vi "ExportMeasuresToHTML.vi"(8 "error in (no error)":errorcluster, 11 "Table in":refnum<vi>) -> (0 "error out":errorcluster)   [LabVIEW 2012]
uses:
  GlobalVariables/UserInfos.vi
  GlobalVariables/MeasureExportStrings.vi
  GlobalVariables/MachineInfos.vi
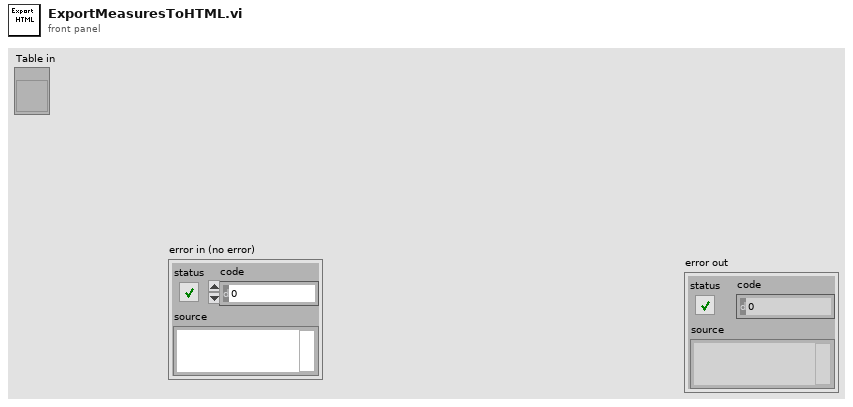
[diagram p1: front panel]
types:
  T1 = enum16{"open", "replace", "create", "open or create", "replace or create", "replace or create with confirmation"}
  T2 = cluster{"SerialNumber":string, "MachineName":string}
  T3 = cluster{"location":string, "Field":string, "Company":string, "Lab":string, "Operator":string, "Well":string, "Lat/Long":string, "Formation":string, "Country":string, "Client":string}
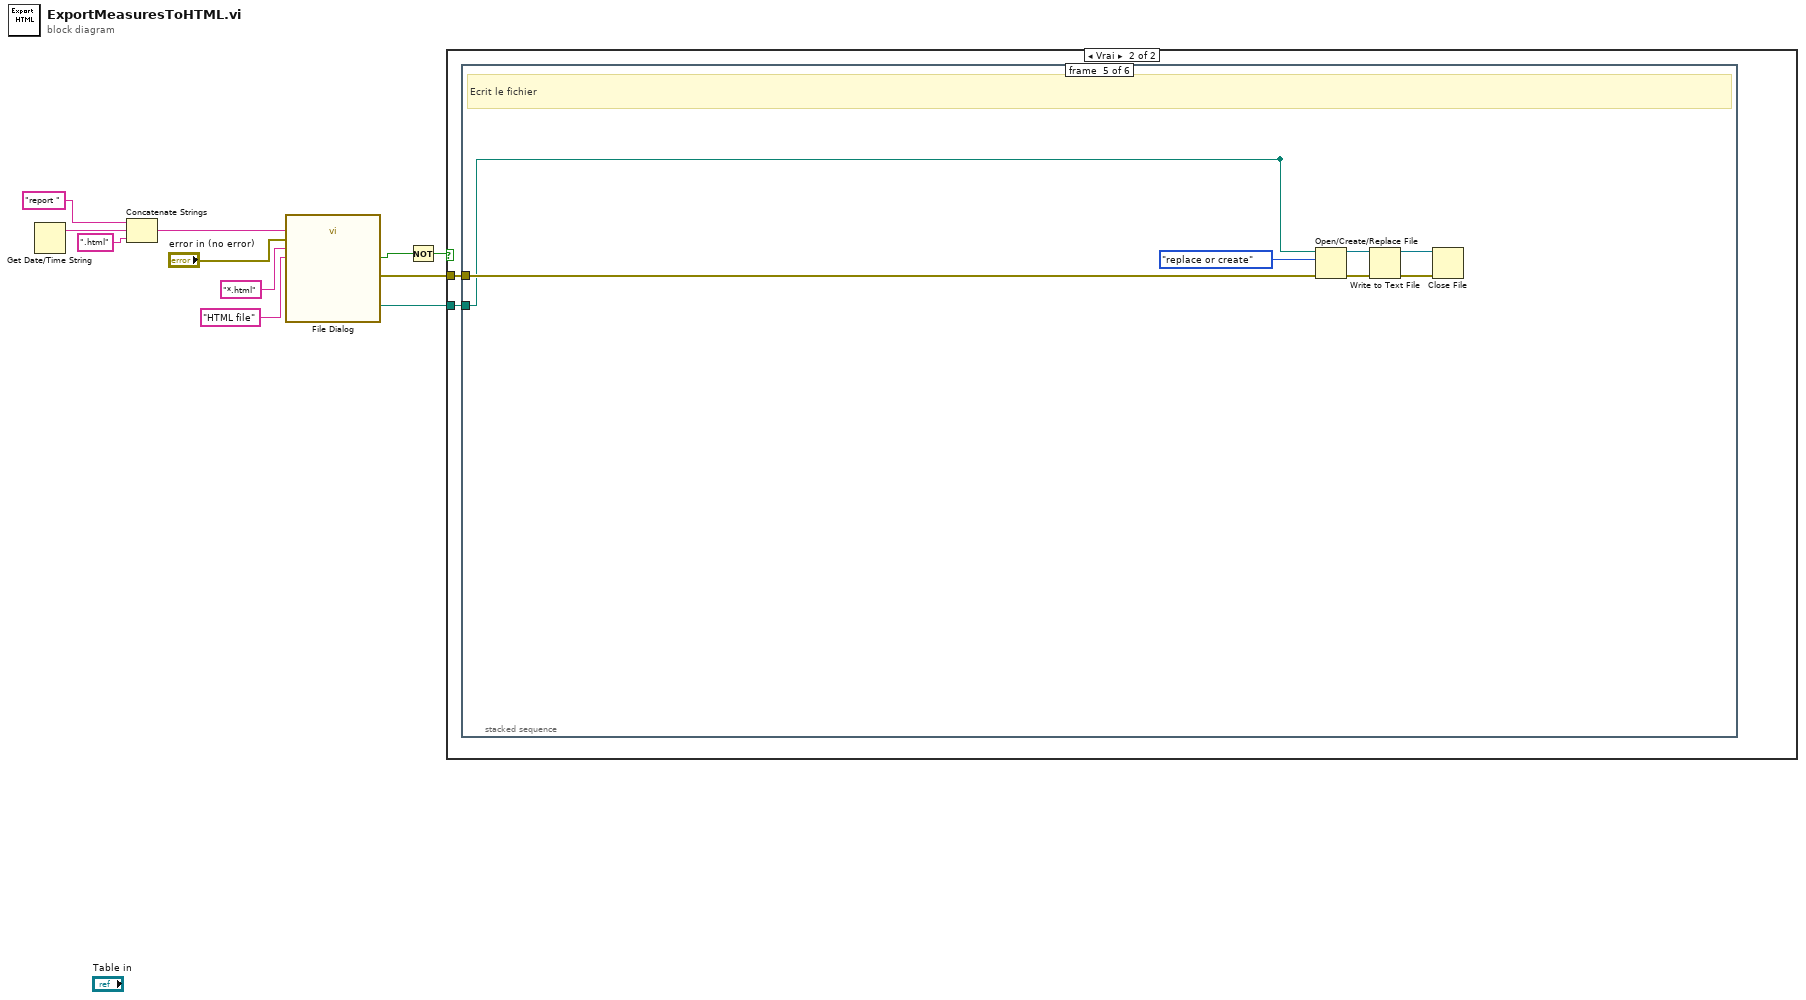
[diagram p0: block diagram]
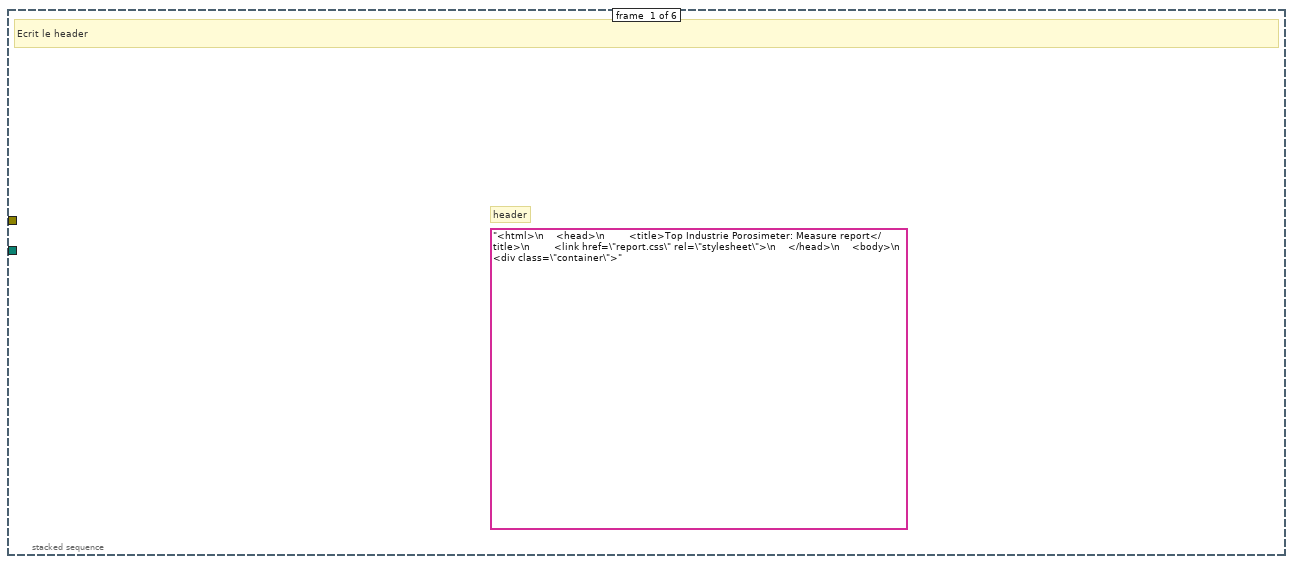
[diagram p3: hidden frame]
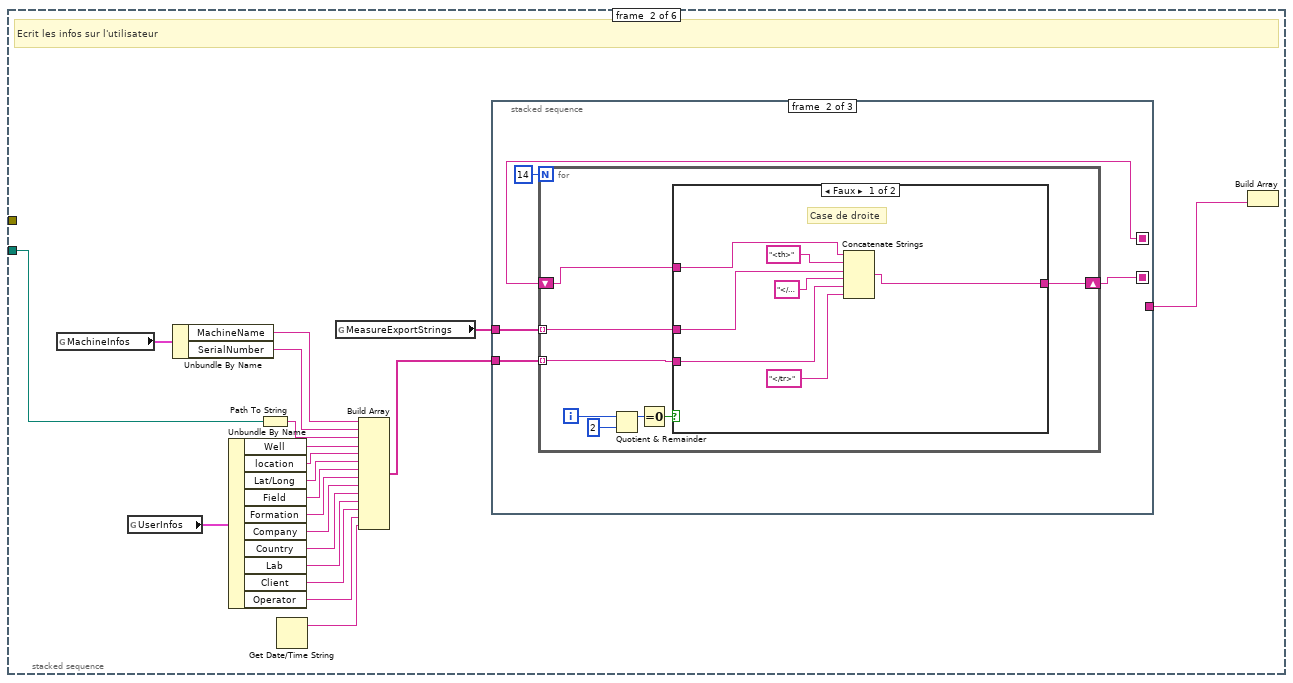
[diagram p4: hidden frame]
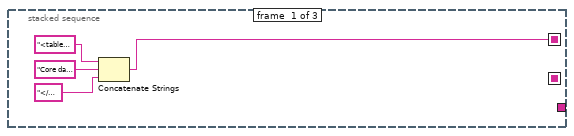
[diagram p5: hidden frame]
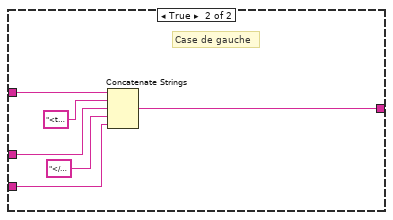
[diagram p6: hidden frame]
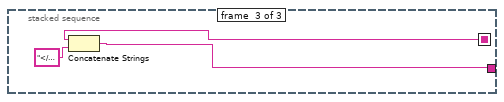
[diagram p7: hidden frame]
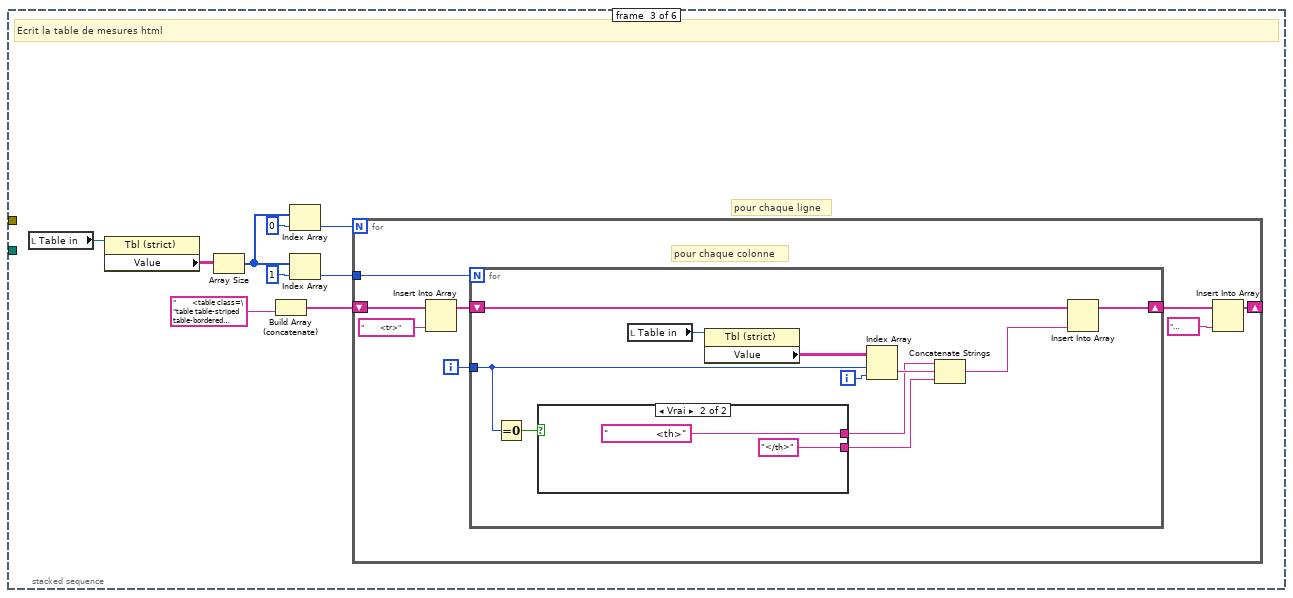
[diagram p8: hidden frame]
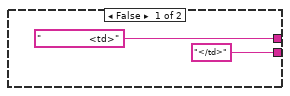
[diagram p9: hidden frame]
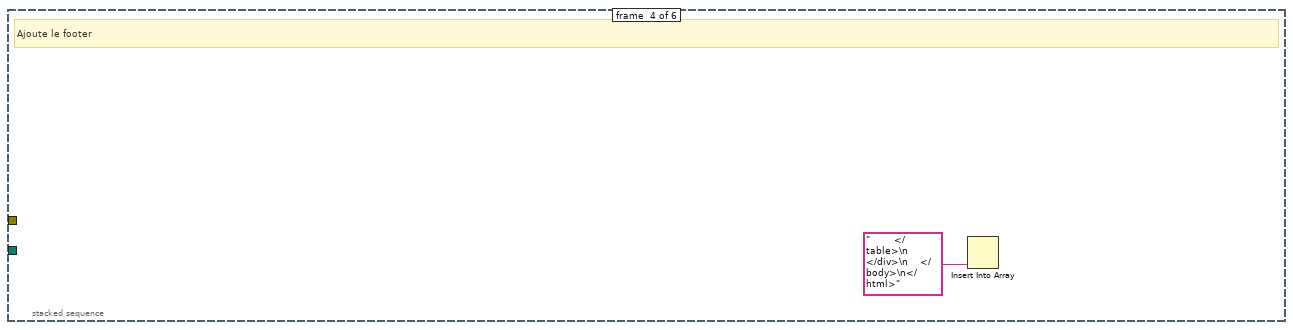
[diagram p10: hidden frame]
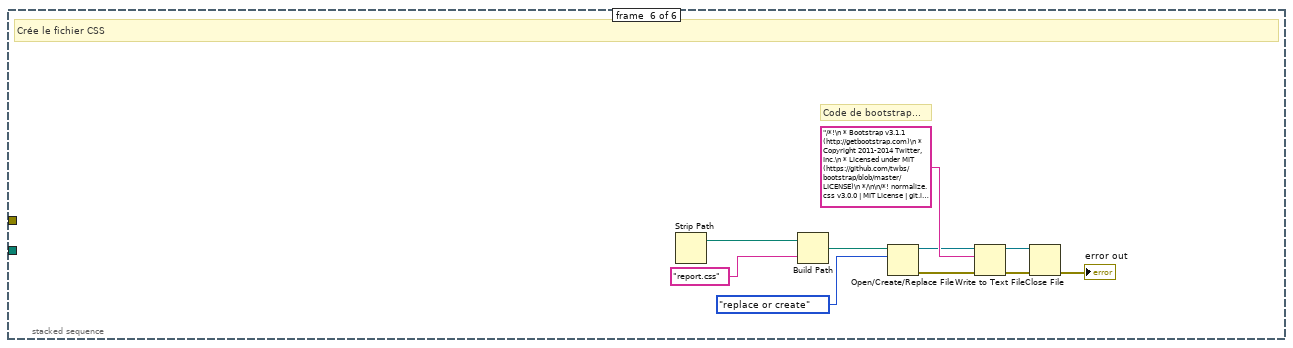
[diagram p11: hidden frame]
diagram:
  n1 = Get Date/Time String() -> (date string=w3:string)  [unwired: 3 in, 1 out]
  n2 = Concatenate Strings("report " ("string"), w3, ".html" ("string")) -> (w4:string)
  n3 = call "File Dialog"("default name"=w4, "error in"="error in (no error)", "pattern (all files)"="*.html", "pattern label"="HTML file") -> ("selected path"=w7:path, "cancelled"=w1:bool, "error out"=w8:errorcluster)  [unwired: 8 in, 1 out]
  n4 = Not(x=w1) -> (.not. x?=w2:bool)
  n5 = case shown="Vrai" w2 {
    tunnel: w8 -> [_ w13]
    tunnel: w7 -> [_ w12]
    frame False {
    }
    frame True {
      n6 = stacked-sequence {
        seq-local: ["<html>\n    <head>\n        <title>Top Industrie Porosimeter: Measure report</title>\n        <link href=\"report.css\" rel=\"stylesheet\">\n    </head>\n    <body>\n    <div class=\"container\">" _ _ _ _ _] -> [_ w36 _ _ _ _]
        seq-local: [_ w35 _ _ _ _] -> [_ _ w78 _ _ _]
        seq-local: [_ _ w77 _ _ _] -> [_ _ _ w105 _ _]
        seq-local: [_ _ _ w104 _ _] -> [_ _ _ _ w112 _]
        seq-local: [_ _ _ _ w113 _] -> [_ _ _ _ _ w120]
        seq-local: [_ _ _ _ w107 _] -> [_ _ _ _ _ w116]
        tunnel: w13 -> [_ _ _ _ w108 _]
        tunnel: w12 -> [_ w22 _ _ w107 _]
        frame #0 {
          # "header"
          # "Ecrit le header"
        }
        frame #1 {
          # "Ecrit les infos sur l'utilisateur"
          n7 = global read "MachineInfos.vi" "MachineInfos"() -> (w17:T2)
          n8 = global read "UserInfos.vi" "UserInfos"() -> (w34:T3)
          n9 = Unbundle By Name(w17) -> ("MachineName"=w16:string, "SerialNumber"=w15:string)
          n10 = Unbundle By Name(w34) -> ("Well"=w33:string, "location"=w32:string, "Lat/Long"=w31:string, "Field"=w30:string, "Formation"=w29:string, "Company"=w26:string, "Country"=w28:string, "Lab"=w27:string, "Client"=w25:string, "Operator"=w24:string)
          n11 = Path To String(path=w22) -> (string=w23:string)
          n12 = Get Date/Time String() -> (date string=w20:string)  [unwired: 3 in, 1 out]
          n13 = global read "MeasureExportStrings.vi" "MeasureExportStrings"() -> (w18:string[])
          n14 = Build Array(w16, w15, w23, w33, w32, w31, w30, w29, w26, w28, w27, w25, w24, w20) -> (w19:string[])
          n15 = stacked-sequence {
            seq-local: [w39 _ _] -> [_ w41 _]
            seq-local: [_ w42 _] -> [_ _ w68]
            tunnel: [_ _ w69] -> w21
            tunnel: w18 -> [_ w44 _]
            tunnel: w19 -> [_ w43 _]
            frame #0 {
              n16 = Concatenate Strings("<table class=\"table table-bordered table-condensed\">\n<tr>\n<td colspan=4> <h2 align=center>\n", "Core data report" ("string"), "</h2></td>\n</tr>" ("string")) -> (w39:string)
            }
            frame #1 {
              n17 = for {
                N: 14 -> [_]
                tunnel: w44 -> [w49] mode=indexing
                tunnel: w43 -> [w48] mode=indexing
                shift-right: [w47] -> w42
                shift-left: w41 -> [w46]
                i -> [w53]
                n18 = Quotient & Remainder(x=w53, y=2) -> (x-y*floor(x/y)=w50:i32)  [unwired: 1 out]
                n19 = Equal To 0?(x=w50) -> (x = 0?=w51:bool)
                n20 = case shown="Faux" w51 {
                  tunnel: w49 -> [w58 w65]
                  tunnel: w48 -> [w57 w63]
                  tunnel: [w55 w62] -> w47
                  tunnel: w46 -> [w54 w61]
                  frame False {
                    # "Case de droite"
                    n21 = Concatenate Strings(w54, "<th>", w58, "</th><td>", w57, "</tr>" ("string")) -> (w55:string)
                  }
                  frame True {
                    # "Case de gauche"
                    n22 = Concatenate Strings(w61, "<tr>\n<th>", w65, "</th><td>", w63) -> (w62:string)
                  }
                }
              }
            }
            frame #2 {
              n23 = Concatenate Strings(w68, "</table>\n" ("string")) -> (w69:string)
            }
          }
          n24 = Build Array(w36, w21) -> (w35:string[])
        }
        frame #2 {
          # "pour chaque ligne"
          # "Ecrit la table de mesures html"
          n25 = local read "Table in"() -> (w74:refnum<vi>)
          n26 = property on="Property Node" class="Tbl (strict)"(reference=w74) -> ("Value"=w75:string[][])  [unwired: 1 in, 2 out]
          n27 = Array Size(array=w75) -> (size(s)=w70:i32[])
          n28 = Build Array (concatenate)(w78, "        <table class=\"table table-striped table-bordered table-responsive\" >") -> (w80:string[])
          n29 = Index Array(array=w70, index=0) -> (element=w73:i32)
          n30 = Index Array(array=w70, index=1) -> (element=w72:i32)
          n31 = for {
            N: w73 -> [_]
            shift-right: [w88] -> w77
            shift-left: w80 -> [w87]
            tunnel: w72 -> [w86]
            i -> [w82]
            # "pour chaque colonne"
            n32 = Insert Into Array(array=w87, new element="        <tr>" ("new element/subarray")) -> (w84:string[])  [unwired: 1 in]
            n33 = for {
              N: w86 -> [_]
              shift-right: [w98] -> w85
              shift-left: w84 -> [w99]
              tunnel: w82 -> [w89]
              i -> [w91]
              n34 = Equal To 0?(x=w89) -> (x = 0?=w90:bool)
              n35 = case shown="Vrai" w90 {
                tunnel: ["</td>" "</th>"] -> w94
                tunnel: ["                <td>" "                <th>"] -> w92
                frame False {
                }
                frame True {
                }
              }
              n36 = local read "Table in"() -> (w95:refnum<vi>)
              n37 = property on="Property Node" class="Tbl (strict)"(reference=w95) -> ("Value"=w97:string[][])  [unwired: 1 in, 2 out]
              n38 = Index Array(array=w97, index (row)=w89, index (col)=w91) -> (element=w96:string)
              n39 = Concatenate Strings(w92, w96, w94) -> (w93:string)
              n40 = Insert Into Array(array=w99, new element=w93) -> (w98:string[])  [unwired: 1 in]
            }
            n41 = Insert Into Array(array=w85, new element="            </tr>") -> (w88:string[])  [unwired: 1 in]
          }
        }
        frame #3 {
          # "Ajoute le footer"
          n42 = Insert Into Array(array=w105, new element="        </table>\n        </div>\n    </body>\n</html>") -> (w104:string[])  [unwired: 1 in]
        }
        frame #4 {
          # "Ecrit le fichier"
          n43 = Open/Create/Replace File(file path (use dialog)=w107, error in=w108, operation (0:open)=T1."replace or create") -> (refnum out=w111:refnum<file>, error out=w114:errorcluster)  [unwired: 3 in, 1 out]
          n44 = Write to Text File(file (use dialog)=w111, text=w112, error in=w114) -> (refnum out=w109:refnum<file>, error out=w115:errorcluster)  [unwired: 1 in, 1 out]
          n45 = Close File(refnum=w109, error in=w115) -> (error out=w113:errorcluster)  [unwired: 1 out]
        }
        frame #5 {
          # "Code de bootstrap..."
          # "Crée le fichier CSS"
          n46 = Strip Path(path=w116) -> (stripped path=w119:path)  [unwired: 1 out]
          n47 = Build Path(base path=w119, name or relative path="report.css") -> (appended path=w117:path)
          n48 = Open/Create/Replace File(file path (use dialog)=w117, error in=w120, operation (0:open)=T1."replace or create") -> (refnum out=w125:refnum<file>, error out=w123:errorcluster)  [unwired: 3 in, 1 out]
          n49 = Write to Text File(file (use dialog)=w125, text="/*!\n * Bootstrap v3.1.1 (http://getbootstrap.com)\n * Copyright 2011-2014 Twitter, Inc.\n * Licensed under MIT (https://github.com/twbs/bootstrap/blob/master/LICENSE)\n */\n\n/*! normalize.css v3.0.0 | MIT License | git.io/normalize */\nhtml {\n  font-family: sans-serif;\n  -webkit-text-size-adjust: 100%;\n      -ms-text-size-adjust: 100%;\n}\nbody {\n  margin: 0;\n}\narticle,\naside,\ndetails,\nfigcaption,\nfigure,\nfooter,\nheader,\nhgroup,\nmain,\nnav,\nsection,\nsummary {\n  display: block;\n}\naudio,\ncanvas,\nprogress,\nvideo {\n  display: inline-block;\n  vertical-align: baseline;\n}\naudio:not([controls]) {\n  display: none;\n  height: 0;\n}\n[hidden],\ntemplate {\n  display: none;\n}\na {\n  background: transparent;\n}\na:active,\na:hover {\n  outline: 0;\n}\nabbr[title] {\n  border-bottom: 1px dotted;\n}\nb,\nstrong {\n  font-weight: bold;\n}\ndfn {\n  font-style: italic;\n}\nh1 {\n  margin: .67em 0;\n  font-size: 2em;\n}\nmark {\n  color: #000;\n  background: #ff0;\n}\nsmall {\n  font-size: 80%;\n}\nsub,\nsup {\n  position: relative;\n  font-size: 75%;\n  line-height: 0;\n  vertical-align: baseline;\n}\nsup {\n  top: -.5em;\n}\nsub {\n  bottom: -.25em;\n}\nimg {\n  border: 0;\n}\nsvg:not(:root) {\n  overflow: hidden;\n}\nfigure {\n  margin: 1em 40px;\n}\nhr {\n  height: 0;\n  -moz-box-sizing: content-box;\n       box-sizing: content-box;\n}\npre {\n  overflow: auto;\n}\ncode,\nkbd,\npre,\nsamp {\n  font-family: monospace, monospace;\n  font-size: 1em;\n}\nbutton,\ninput,\noptgroup,\nselect,\ntextarea {\n  margin: 0;\n  font: inherit;\n  color: inherit;\n}\nbutton {\n  overflow: visible;\n}\nbutton,\nselect {\n  text-transform: none;\n}\nbutton,\nhtml input[type=\"button\"],\ninput[type=\"reset\"],\ninput[type=\"submit\"] {\n  -webkit-appearance: button;\n  cursor: pointer;\n}\nbutton[disabled],\nhtml input[disabled] {\n  cursor: default;\n}\nbutton::-moz-focus-inner,\ninput::-moz-focus-inner {\n  padding: 0;\n  border: 0;\n}\ninput {\n  line-height: normal;\n}\ninput[type=\"checkbox\"],\ninput[type=\"radio\"] {\n  box-sizing: border-box;\n  padding: 0;\n}\ninput[type=\"number\"]::-webkit-inner-spin-button,\ninput[type=\"number\"]::-webkit-outer-spin-button {\n  height: auto;\n}\ninput[type=\"search\"] {\n  -webkit-box-sizing: content-box;\n     -moz-box-sizing: content-box;\n          box-sizing: content-box;\n  -webkit-appearance: textfield;\n}\ninput[type=\"search\"]::-webkit-search-cancel-button,\ninput[type=\"search\"]::-webkit-search-decoration {\n  -webkit-appearance: none;\n}\nfieldset {\n  padding: .35em .625em .75em;\n  margin: 0 2px;\n  border: 1px solid #c0c0c0;\n}\nlegend {\n  padding: 0;\n  border: 0;\n}\ntextarea {\n  overflow: auto;\n}\noptgroup {\n  font-weight: bold;\n}\ntable {\n  border-spacing: 0;\n  border-collapse: collapse;\n}\ntd,\nth {\n  padding: 0;\n}\n@media print {\n  * {\n    color: #000 !important;\n    text-shadow: none !important;\n    background: transparent !important;\n    box-shadow: none !important;\n  }\n  a,\n  a:visited {\n    text-decoration: underline;\n  }\n  a[href]:after {\n    content: \" (\" attr(href) \")\";\n  }\n  abbr[title]:after {\n    content: \" (\" attr(title) \")\";\n  }\n  a[href^=\"javascript:\"]:after,\n  a[href^=\"#\"]:after {\n    content: \"\";\n  }\n  pre,\n  blockquote {\n    border: 1px solid #999;\n\n    page-break-inside: avoid;\n  }\n  thead {\n    display: table-header-group;\n  }\n  tr,\n  img {\n    page-break-inside: avoid;\n  }\n  img {\n    max-width: 100% !important;\n  }\n  p,\n  h2,\n  h3 {\n    orphans: 3;\n    widows: 3;\n  }\n  h2,\n  h3 {\n    page-break-after: avoid;\n  }\n  select {\n    background: #fff !important;\n  }\n  .navbar {\n    display: none;\n  }\n  .table td,\n  .table th {\n    background-color: #fff !important;\n  }\n  .btn > .caret,\n  .dropup > .btn > .caret {\n    border-top-color: #000 !important;\n  }\n  .label {\n    border: 1px solid #000;\n  }\n  .table {\n    border-collapse: collapse !important;\n  }\n  .table-bordered th,\n  .table-bordered td {\n    border: 1px solid #ddd !important;\n  }\n}\n* {\n  -webkit-box-sizing: border-box;\n     -moz-box-sizing: border-box;\n          box-sizing: border-box;\n}\n*:before,\n*:after {\n  -webkit-box-sizing: border-box;\n     -moz-box-sizing: border-box;\n          box-sizing: border-box;\n}\nhtml {\n  font-size: 62.5%;\n\n  -webkit-tap-highlight-color: rgba(0, 0, 0, 0);\n}\nbody {\n  font-family: \"Helvetica Neue\", Helvetica, Arial, sans-serif;\n  font-size: 14px;\n  line-height: 1.42857143;\n  color: #333;\n  background-color: #fff;\n}\ninput,\nbutton,\nselect,\ntextarea {\n  font-family: inherit;\n  font-size: inherit;\n  line-height: inherit;\n}\na {\n  color: #428bca;\n  text-decoration: none;\n}\na:hover,\na:focus {\n  color: #2a6496;\n  text-decoration: underline;\n}\na:focus {\n  outline: thin dotted;\n  outline: 5px auto -webkit-focus-ring-color;\n  outline-offset: -2px;\n}\nfigure {\n  margin: 0;\n}\nimg {\n  vertical-align: middle;\n}\n.img-responsive,\n.thumbnail > img,\n.thumbnail a > img,\n.carousel-inner > .item > img,\n.carousel-inner > .item > a > img {\n  display: block;\n  max-width: 100%;\n  height: auto;\n}\n.img-rounded {\n  border-radius: 6px;\n}\n.img-thumbnail {\n  display: inline-block;\n  max-width: 100%;\n  height: auto;\n  padding: 4px;\n  line-height: 1.42857143;\n  background-color: #fff;\n  border: 1px solid #ddd;\n  border-radius: 4px;\n  -webkit-transition: all .2s ease-in-out;\n          transition: all .2s ease-in-out;\n}\n.img-circle {\n  border-radius: 50%;\n}\nhr {\n  margin-top: 20px;\n  margin-bottom: 20px;\n  border: 0;\n  border-top: 1px solid #eee;\n}\n.sr-only {\n  position: absolute;\n  width: 1px;\n  height: 1px;\n  padding: 0;\n  margin: -1px;\n  overflow: hidden;\n  clip: rect(0, 0, 0, 0);\n  border: 0;\n}\nh1,\nh2,\nh3,\nh4,\nh5,\nh6,\n.h1,\n.h2,\n.h3,\n.h4,\n.h5,\n.h6 {\n  font-family: inherit;\n  font-weight: 500;\n  line-height: 1.1;\n  color: inherit;\n}\nh1 small,\nh2 small,\nh3 small,\nh4 small,\nh5 small,\nh6 small,\n.h1 small,\n.h2 small,\n.h3 small,\n.h4 small,\n.h5 small,\n.h6 small,\nh1 .small,\nh2 .small,\nh3 .small,\nh4 .small,\nh5 .small,\nh6 .small,\n.h1 .small,\n.h2 .small,\n.h3 .small,\n.h4 .small,\n.h5 .small,\n.h6 .small {\n  font-weight: normal;\n  line-height: 1;\n  color: #999;\n}\nh1,\n.h1,\nh2,\n.h2,\nh3,\n.h3 {\n  margin-top: 20px;\n  margin-bottom: 10px;\n}\nh1 small,\n.h1 small,\nh2 small,\n.h2 small,\nh3 small,\n.h3 small,\nh1 .small,\n.h1 .small,\nh2 .small,\n.h2 .small,\nh3 .small,\n.h3 .small {\n  font-size: 65%;\n}\nh4,\n.h4,\nh5,\n.h5,\nh6,\n.h6 {\n  margin-top: 10px;\n  margin-bottom: 10px;\n}\nh4 small,\n.h4 small,\nh5 small,\n.h5 small,\nh6 small,\n.h6 small,\nh4 .small,\n.h4 .small,\nh5 .small,\n.h5 .small,\nh6 .small,\n.h6 .small {\n  font-size: 75%;\n}\nh1,\n.h1 {\n  font-size: 36px;\n}\nh2,\n.h2 {\n  font-size: 30px;\n}\nh3,\n.h3 {\n  font-size: 24px;\n}\nh4,\n.h4 {\n  font-size: 18px;\n}\nh5,\n.h5 {\n  font-size: 14px;\n}\nh6,\n.h6 {\n  font-size: 12px;\n}\np {\n  margin: 0 0 10px;\n}\n.lead {\n  margin-bottom: 20px;\n  font-size: 16px;\n  font-weight: 200;\n  line-height: 1.4;\n}\n@media (min-width: 768px) {\n  .lead {\n    font-size: 21px;\n  }\n}\nsmall,\n.small {\n  font-size: 85%;\n}\ncite {\n  font-style: normal;\n}\n.text-left {\n  text-align: left;\n}\n.text-right {\n  text-align: right;\n}\n.text-center {\n  text-align: center;\n}\n.text-justify {\n  text-align: justify;\n}\n.text-muted {\n  color: #999;\n}\n.text-primary {\n  color: #428bca;\n}\na.text-primary:hover {\n  color: #3071a9;\n}\n.text-success {\n  color: #3c763d;\n}\na.text-success:hover {\n  color: #2b542c;\n}\n.text-info {\n  color: #31708f;\n}\na.text-info:hover {\n  color: #245269;\n}\n.text-warning {\n  color: #8a6d3b;\n}\na.text-warning:hover {\n  color: #66512c;\n}\n.text-danger {\n  color: #a94442;\n}\na.text-danger:hover {\n  color: #843534;\n}\n.bg-primary {\n  color: #fff;\n  background-color: #428bca;\n}\na.bg-primary:hover {\n  background-color: #3071a9;\n}\n.bg-success {\n  background-color: #dff0d8;\n}\na.bg-success:hover {\n  background-color: #c1e2b3;\n}\n.bg-info {\n  background-color: #d9edf7;\n}\na.bg-info:hover {\n  background-color: #afd9ee;\n}\n.bg-warning {\n  background-color: #fcf8e3;\n}\na.bg-warning:hover {\n  background-color: #f7ecb5;\n}\n.bg-danger {\n  background-color: #f2dede;\n}\na.bg-danger:hover {\n  background-color: #e4b9b9;\n}\n.page-header {\n  padding-bottom: 9px;\n  margin: 40px 0 20px;\n  border-bottom: 1px solid #eee;\n}\nul,\nol {\n  margin-top: 0;\n  margin-bottom: 10px;\n}\nul ul,\nol ul,\nul ol,\nol ol {\n  margin-bottom: 0;\n}\n.list-unstyled {\n  padding-left: 0;\n  list-style: none;\n}\n.list-inline {\n  padding-left: 0;\n  margin-left: -5px;\n  list-style: none;\n}\n.list-inline > li {\n  display: inline-block;\n  padding-right: 5px;\n  padding-left: 5px;\n}\ndl {\n  margin-top: 0;\n  margin-bottom: 20px;\n}\ndt,\ndd {\n  line-height: 1.42857143;\n}\ndt {\n  font-weight: bold;\n}\ndd {\n  margin-left: 0;\n}\n@media (min-width: 768px) {\n  .dl-horizontal dt {\n    float: left;\n    width: 160px;\n    overflow: hidden;\n    clear: left;\n    text-align: right;\n    text-overflow: ellipsis;\n    white-space: nowrap;\n  }\n  .dl-horizontal dd {\n    margin-left: 180px;\n  }\n}\nabbr[title],\nabbr[data-original-title] {\n  cursor: help;\n  border-bottom: 1px dotted #999;\n}\n.initialism {\n  font-size: 90%;\n  text-transform: uppercase;\n}\nblockquote {\n  padding: 10px 20px;\n  margin: 0 0 20px;\n  font-size: 17.5px;\n  border-left: 5px solid #eee;\n}\nblockquote p:last-child,\nblockquote ul:last-child,\nblockquote ol:last-child {\n  margin-bottom: 0;\n}\nblockquote footer,\nblockquote small,\nblockquote .small {\n  display: block;\n  font-size: 80%;\n  line-height: 1.42857143;\n  color: #999;\n}\nblockquote footer:before,\nblockquote small:before,\nblockquote .small:before {\n  content: '\\2014 \\00A0';\n}\n.blockquote-reverse,\nblockquote.pull-right {\n  padding-right: 15px;\n  padding-left: 0;\n  text-align: right;\n  border-right: 5px solid #eee;\n  border-left: 0;\n}\n.blockquote-reverse footer:before,\nblockquote.pull-right footer:before,\n.blockquote-reverse small:before,\nblockquote.pull-right small:before,\n.blockquote-reverse .small:before,\nblockquote.pull-right .small:before {\n  content: '';\n}\n.blockquote-reverse footer:after,\nblockquote.pull-right footer:after,\n.blockquote-reverse small:after,\nblockquote.pull-right small:after,\n.blockquote-reverse .small:after,\nblockquote.pull-right .small:after {\n  content: '\\00A0 \\2014';\n}\nblockquote:before,\nblockquote:after {\n  content: \"\";\n}\naddress {\n  margin-bottom: 20px;\n  font-style: normal;\n  line-height: 1.42857143;\n}\ncode,\nkbd,\npre,\nsamp {\n  font-family: Menlo, Monaco, Consolas, \"Courier New\", monospace;\n}\ncode {\n  padding: 2px 4px;\n  font-size: 90%;\n  color: #c7254e;\n  white-space: nowrap;\n  background-color: #f9f2f4;\n  border-radius: 4px;\n}\nkbd {\n  padding: 2px 4px;\n  font-size: 90%;\n  color: #fff;\n  background-color: #333;\n  border-radius: 3px;\n  box-shadow: inset 0 -1px 0 rgba(0, 0, 0, .25);\n}\npre {\n  display: block;\n  padding: 9.5px;\n  margin: 0 0 10px;\n  font-size: 13px;\n  line-height: 1.42857143;\n  color: #333;\n  word-break: break-all;\n  word-wrap: break-word;\n  background-color: #f5f5f5;\n  border: 1px solid #ccc;\n  border-radius: 4px;\n}\npre code {\n  padding: 0;\n  font-size: inherit;\n  color: inherit;\n  white-space: pre-wrap;\n  background-color: transparent;\n  border-radius: 0;\n}\n.pre-scrollable {\n  max-height: 340px;\n  overflow-y: scroll;\n}\n.container {\n  padding-right: 15px;\n  padding-left: 15px;\n  margin-right: auto;\n  margin-left: auto;\n}\n@media (min-width: 768px) {\n  .container {\n    width: 750px;\n  }\n}\n@media (min-width: 992px) {\n  .container {\n    width: 970px;\n  }\n}\n@media (min-width: 1200px) {\n  .container {\n    width: 1170px;\n  }\n}\n.container-fluid {\n  padding-right: 15px;\n  padding-left: 15px;\n  margin-right: auto;\n  margin-left: auto;\n}\n.row {\n  margin-right: -15px;\n  margin-left: -15px;\n}\n.col-xs-1, .col-sm-1, .col-md-1, .col-lg-1, .col-xs-2, .col-sm-2, .col-md-2, .col-lg-2, .col-xs-3, .col-sm-3, .col-md-3, .col-lg-3, .col-xs-4, .col-sm-4, .col-md-4, .col-lg-4, .col-xs-5, .col-sm-5, .col-md-5, .col-lg-5, .col-xs-6, .col-sm-6, .col-md-6, .col-lg-6, .col-xs-7, .col-sm-7, .col-md-7, .col-lg-7, .col-xs-8, .col-sm-8, .col-md-8, .col-lg-8, .col-xs-9, .col-sm-9, .col-md-9, .col-lg-9, .col-xs-10, .col-sm-10, .col-md-10, .col-lg-10, .col-xs-11, .col-sm-11, .col-md-11, .col-lg-11, .col-xs-12, .col-sm-12, .col-md-12, .col-lg-12 {\n  position: relative;\n  min-height: 1px;\n  padding-right: 15px;\n  padding-left: 15px;\n}\n.col-xs-1, .col-xs-2, .col-xs-3, .col-xs-4, .col-xs-5, .col-xs-6, .col-xs-7, .col-xs-8, .col-xs-9, .col-xs-10, .col-xs-11, .col-xs-12 {\n  float: left;\n}\n.col-xs-12 {\n  width: 100%;\n}\n.col-xs-11 {\n  width: 91.66666667%;\n}\n.col-xs-10 {\n  width: 83.33333333%;\n}\n.col-xs-9 {\n  width: 75%;\n}\n.col-xs-8 {\n  width: 66.66666667%;\n}\n.col-xs-7 {\n  width: 58.33333333%;\n}\n.col-xs-6 {\n  width: 50%;\n}\n.col-xs-5 {\n  width: 41.66666667%;\n}\n.col-xs-4 {\n  width: 33.33333333%;\n}\n.col-xs-3 {\n  width: 25%;\n}\n.col-xs-2 {\n  width: 16.66666667%;\n}\n.col-xs-1 {\n  width: 8.33333333%;\n}\n.col-xs-pull-12 {\n  right: 100%;\n}\n.col-xs-pull-11 {\n  right: 91.66666667%;\n}\n.col-xs-pull-10 {\n  right: 83.33333333%;\n}\n.col-xs-pull-9 {\n  right: 75%;\n}\n.col-xs-pull-8 {\n  right: 66.66666667%;\n}\n.col-xs-pull-7 {\n  right: 58.33333333%;\n}\n.col-xs-pull-6 {\n  right: 50%;\n}\n.col-xs-pull-5 {\n  right: 41.66666667%;\n}\n.col-xs-pull-4 {\n  right: 33.33333333%;\n}\n.col-xs-pull-3 {\n  right: 25%;\n}\n.col-xs-pull-2 {\n  right: 16.66666667%;\n}\n.col-xs-pull-1 {\n  right: 8.33333333%;\n}\n.col-xs-pull-0 {\n  right: 0;\n}\n.col-xs-push-12 {\n  left: 100%;\n}\n.col-xs-push-11 {\n  left: 91.66666667%;\n}\n.col-xs-push-10 {\n  left: 83.33333333%;\n}\n.col-xs-push-9 {\n  left: 75%;\n}\n.col-xs-push-8 {\n  left: 66.66666667%;\n}\n.col-xs-push-7 {\n  left: 58.33333333%;\n}\n.col-xs-push-6 {\n  left: 50%;\n}\n.col-xs-push-5 {\n  left: 41.66666667%;\n}\n.col-xs-push-4 {\n  left: 33.33333333%;\n}\n.col-xs-push-3 {\n  left: 25%;\n}\n.col-xs-push-2 {\n  left: 16.66666667%;\n}\n.col-xs-push-1 {\n  left: 8.33333333%;\n}\n.col-xs-push-0 {\n  left: 0;\n}\n.col-xs-offset-12 {\n  margin-left: 100%;\n}\n.col-xs-offset-11 {\n  margin-left: 91.66666667%;\n}\n.col-xs-offset-10 {\n  margin-left: 83.33333333%;\n}\n.col-xs-offset-9 {\n  margin-left: 75%;\n}\n.col-xs-offset-8 {\n  margin-left: 66.66666667%;\n}\n.col-xs-offset-7 {\n  margin-left: 58.33333333%;\n}\n.col-xs-offset-6 {\n  margin-left: 50%;\n}\n.col-xs-offset-5 {\n  margin-left: 41.66666667%;\n}\n.col-xs-offset-4 {\n  margin-left: 33.33333333%;\n}\n.col-xs-offset-3 {\n  margin-left: 25%;\n}\n.col-xs-offset-2 {\n  margin-left: 16.66666667%;\n}\n.col-xs-offset-1 {\n  margin-left: 8.33333333%;\n}\n.col-xs-offset-0 {\n  margin-left: 0;\n}\n@media (min-width: 768px) {\n  .col-sm-1, .col-sm-2, .col-sm-3, .col-sm-4, .col-sm-5, .col-sm-6, .col-sm-7, .col-sm-8, .col-sm-9, .col-sm-10, .col-sm-11, .col-sm-12 {\n    float: left;\n  }\n  .col-sm-12 {\n    width: 100%;\n  }\n  .col-sm-11 {\n    width: 91.66666667%;\n  }\n  .col-sm-10 {\n    width: 83.33333333%;\n  }\n  .col-sm-9 {\n    width: 75%;\n  }\n  .col-sm-8 {\n    width: 66.66666667%;\n  }\n  .col-sm-7 {\n    width: 58.33333333%;\n  }\n  .col-sm-6 {\n    width: 50%;\n  }\n  .col-sm-5 {\n    width: 41.66666667%;\n  }\n  .col-sm-4 {\n    width: 33.33333333%;\n  }\n  .col-sm-3 {\n    width: 25%;\n  }\n  .col-sm-2 {\n    width: 16.66666667%;\n  }\n  .col-sm-1 {\n    width: 8.33333333%;\n  }\n  .col-sm-pull-12 {\n    right: 100%;\n  }\n  .col-sm-pull-11 {\n    right: 91.66666667%;\n  }\n  .col-sm-pull-10 {\n    right: 83.33333333%;\n  }\n  .col-sm-pull-9 {\n    right: 75%;\n  }\n  .col-sm-pull-8 {\n    right: 66.66666667%;\n  }\n  .col-sm-pull-7 {\n    right: 58.33333333%;\n  }\n  .col-sm-pull-6 {\n    right: 50%;\n  }\n  .col-sm-pull-5 {\n    right: 41.66666667%;\n  }\n  .col-sm-pull-4 {\n    right: 33.33333333%;\n  }\n  .col-sm-pull-3 {\n    right: 25%;\n  }\n  .col-sm-pull-2 {\n    right: 16.66666667%;\n  }\n  .col-sm-pull-1 {\n    right: 8.33333333%;\n  }\n  .col-sm-pull-0 {\n    right: 0;\n  }\n  .col-sm-push-12 {\n    left: 100%;\n  }\n  .col-sm-push-11 {\n    left: 91.66666667%;\n  }\n  .col-sm-push-10 {\n    left: 83.33333333%;\n  }\n  .col-sm-push-9 {\n    left: 75%;\n  }\n  .col-sm-push-8 {\n    left: 66.66666667%;\n  }\n  .col-sm-push-7 {\n    left: 58.33333333%;\n  }\n  .col-sm-push-6 {\n    left: 50%;\n  }\n  .col-sm-push-5 {\n    left: 41.66666667%;\n  }\n  .col-sm-push-4 {\n    left: 33.33333333%;\n  }\n  .col-sm-push-3 {\n    left: 25%;\n  }\n  .col-sm-push-2 {\n    left: 16.66666667%;\n  }\n  .col-sm-push-1 {\n    left: 8.33333333%;\n  }\n  .col-sm-push-0 {\n    left: 0;\n  }\n  .col-sm-offset-12 {\n    margin-left: 100%;\n  }\n  .col-sm-offset-11 {\n    margin-left: 91.66666667%;\n  }\n  .col-sm-offset-10 {\n    margin-left: 83.33333333%;\n  }\n  .col-sm-offset-9 {\n    margin-left: 75%;\n  }\n  .col-sm-offset-8 {\n    margin-left: 66.66666667%;\n  }\n  .col-sm-offset-7 {\n    margin-left: 58.33333333%;\n  }\n  .col-sm-offset-6 {\n    margin-left: 50%;\n  }\n  .col-sm-offset-5 {\n    margin-left: 41.66666667%;\n  }\n  .col-sm-offset-4 {\n    margin-left: 33.33333333%;\n  }\n  .col-sm-offset-3 {\n    margin-left: 25%;\n  }\n  .col-sm-offset-2 {\n    margin-left: 16.66666667%;\n  }\n  .col-sm-offset-1 {\n    margin-left: 8.33333333%;\n  }\n  .col-sm-offset-0 {\n    margin-left: 0;\n  }\n}\n@media (min-width: 992px) {\n  .col-md-1, .col-md-2, .col-md-3, .col-md-4, .col-md-5, .col-md-6, .col-md-7, .col-md-8, .col-md-9, .col-md-10, .col-md-11, .col-md-12 {\n    float: left;\n  }\n  .col-md-12 {\n    width: 100%;\n  }\n  .col-md-11 {\n    width: 91.66666667%;\n  }\n  .col-md-10 {\n    width: 83.33333333%;\n  }\n  .col-md-9 {\n    width: 75%;\n  }\n  .col-md-8 {\n    width: 66.66666667%;\n  }\n  .col-md-7 {\n    width: 58.33333333%;\n  }\n  .col-md-6 {\n    width: 50%;\n  }\n  .col-md-5 {\n    width: 41.66666667%;\n  }\n  .col-md-4 {\n    width: 33.33333333%;\n  }\n  .col-md-3 {\n    width: 25%;\n  }\n  .col-md-2 {\n    width: 16.66666667%;\n  }\n  .col-md-1 {\n    width: 8.33333333%;\n  }\n  .col-md-pull-12 {\n    right: 100%;\n  }\n  .col-md-pull-11 {\n    right: 91.66666667%;\n  }\n  .col-md-pull-10 {\n    right: 83.33333333%;\n  }\n  .col-md-pull-9 {\n    right: 75%;\n  }\n  .col-md-pull-8 {\n    right: 66.66666667%;\n  }\n  .col-md-pull-7 {\n    right: 58.33333333%;\n  }\n  .col-md-pull-6 {\n    right: 50%;\n  }\n  .col-md-pull-5 {\n    right: 41.66666667%;\n  }\n  .col-md-pull-4 {\n    right: 33.33333333%;\n  }\n  .col-md-pull-3 {\n    right: 25%;\n  }\n  .col-md-pull-2 {\n    right: 16.66666667%;\n  }\n  .col-md-pull-1 {\n    right: 8.33333333%;\n  }\n  .col-md-pull-0 {\n    right: 0;\n  }\n  .col-md-push-12 {\n    left: 100%;\n  }\n  .col-md-push-11 {\n    left: 91.66666667%;\n  }\n  .col-md-push-10 {\n    left: 83.33333333%;\n  }\n  .col-md-push-9 {\n    left: 75%;\n  }\n  .col-md-push-8 {\n    left: 66.66666667%;\n  }\n  .col-md-push-7 {\n    left: 58.33333333%;\n  }\n  .col-md-push-6 {\n    left: 50%;\n  }\n  .col-md-push-5 {\n    left: 41.66666667%;\n  }\n  .col-md-push-4 {\n    left: 33.33333333%;\n  }\n  .col-md-push-3 {\n    left: 25%;\n  }\n  .col-md-push-2 {\n    left: 16.66666667%;\n  }\n  .col-md-push-1 {\n    left: 8.33333333%;\n  }\n  .col-md-push-0 {\n    left: 0;\n  }\n  .col-md-offset-12 {\n    margin-left: 100%;\n  }\n  .col-md-offset-11 {\n    margin-left: 91.66666667%;\n  }\n  .col-md-offset-10 {\n    margin-left: 83.33333333%;\n  }\n  .col-md-offset-9 {\n    margin-left: 75%;\n  }\n  .col-md-offset-8 {\n    margin-left: 66.66666667%;\n  }\n  .col-md-offset-7 {\n    margin-left: 58.33333333%;\n  }\n  .col-md-offset-6 {\n    margin-left: 50%;\n  }\n  .col-md-offset-5 {\n    margin-left: 41.66666667%;\n  }\n  .col-md-offset-4 {\n    margin-left: 33.33333333%;\n  }\n  .col-md-offset-3 {\n    margin-left: 25%;\n  }\n  .col-md-offset-2 {\n    margin-left: 16.66666667%;\n  }\n  .col-md-offset-1 {\n    margin-left: 8.33333333%;\n  }\n  .col-md-offset-0 {\n    margin-left: 0;\n  }\n}\n@media (min-width: 1200px) {\n  .col-lg-1, .col-lg-2, .col-lg-3, .col-lg-4, .col-lg-5, .col-lg-6, .col-lg-7, .col-lg-8, .col-lg-9, .col-lg-10, .col-lg-11, .col-lg-12 {\n    float: left;\n  }\n  .col-lg-12 {\n    width: 100%;\n  }\n  .col-lg-11 {\n    width: 91.66666667%;\n  }\n  .col-lg-10 {\n    width: 83.33333333%;\n  }\n  .col-lg-9 {\n    width: 75%;\n  }\n  .col-lg-8 {\n    width: 66.66666667%;\n  }\n  .col-lg-7 {\n    width: 58.33333333%;\n  }\n  .col-lg-6 {\n    width: 50%;\n  }\n  .col-lg-5 {\n    width: 41.66666667%;\n  }\n  .col-lg-4 {\n    width: 33.33333333%;\n  }\n  .col-lg-3 {\n    width: 25%;\n  }\n  .col-lg-2 {\n    width: 16.66666667%;\n  }\n  .col-lg-1 {\n    width: 8.33333333%;\n  }\n  .col-lg-pull-12 {\n    right: 100%;\n  }\n  .col-lg-pull-11 {\n    right: 91.66666667%;\n  }\n  .col-lg-pull-10 {\n    right: 83.33333333%;\n  }\n  .col-lg-pull-9 {\n    right: 75%;\n  }\n  .col-lg-pull-8 {\n    right: 66.66666667%;\n  }\n  .col-lg-pull-7 {\n    right: 58.33333333%;\n  }\n  .col-lg-pull-6 {\n    right: 50%;\n  }\n  .col-lg-pull-5 {\n    right: 41.66666667%;\n  }\n  .col-lg-pull-4 {\n    right: 33.33333333%;\n  }\n  .col-lg-pull-3 {\n    right: 25%;\n  }\n  .col-lg-pull-2 {\n    right: 16.66666667%;\n  }\n  .col-lg-pull-1 {\n    right: 8.33333333%;\n  }\n  .col-lg-pull-0 {\n    right: 0;\n  }\n  .col-lg-push-12 {\n    left: 100%;\n  }\n  .col-lg-push-11 {\n    left: 91.66666667%;\n  }\n  .col-lg-push-10 {\n    left: 83.33333333%;\n  }\n  .col-lg-push-9 {\n    left: 75%;\n  }\n  .col-lg-push-8 {\n    left: 66.66666667%;\n  }\n  .col-lg-push-7 {\n    left: 58.33333333%;\n  }\n  .col-lg-push-6 {\n    left: 50%;\n  }\n  .col-lg-push-5 {\n    left: 41.66666667%;\n  }\n  .col-lg-push-4 {\n    left: 33.33333333%;\n  }\n  .col-lg-push-3 {\n    left: 25%;\n  }\n  .col-lg-push-2 {\n    left: 16.66666667%;\n  }\n  .col-lg-push-1 {\n    left: 8.33333333%;\n  }\n  .col-lg-push-0 {\n    left: 0;\n  }\n  .col-lg-offset-12 {\n    margin-left: 100%;\n  }\n  .col-lg-offset-11 {\n    margin-left: 91.66666667%;\n  }\n  .col-lg-offset-10 {\n    margin-left: 83.33333333%;\n  }\n  .col-lg-offset-9 {\n    margin-left: 75%;\n  }\n  .col-lg-offset-8 {\n    margin-left: 66.66666667%;\n  }\n  .col-lg-offset-7 {\n    margin-left: 58.33333333%;\n  }\n  .col-lg-offset-6 {\n    margin-left: 50%;\n  }\n  .col-lg-offset-5 {\n    margin-left: 41.66666667%;\n  }\n  .col-lg-offset-4 {\n    margin-left: 33.33333333%;\n  }\n  .col-lg-offset-3 {\n    margin-left: 25%;\n  }\n  .col-lg-offset-2 {\n    margin-left: 16.66666667%;\n  }\n  .col-lg-offset-1 {\n    margin-left: 8.33333333%;\n  }\n  .col-lg-offset-0 {\n    margin-left: 0;\n  }\n}\ntable {\n  max-width: 100%;\n  background-color: transparent;\n}\nth {\n  text-align: left;\n}\n.table {\n  width: 100%;\n  margin-bottom: 20px;\n}\n.table > thead > tr > th,\n.table > tbody > tr > th,\n.table > tfoot > tr > th,\n.table > thead > tr > td,\n.table > tbody > tr > td,\n.table > tfoot > tr > td {\n  padding: 2px;\n  line-height: 1.42857143;\n  vertical-align: top;\n  border-top: 1px solid #ddd;\n}\n.table > thead > tr > th {\n  vertical-align: bottom;\n  border-bottom: 2px solid #ddd;\n}\n.table > caption + thead > tr:first-child > th,\n.table > colgroup + thead > tr:first-child > th,\n.table > thead:first-child > tr:first-child > th,\n.table > caption + thead > tr:first-child > td,\n.table > colgroup + thead > tr:first-child > td,\n.table > thead:first-child > tr:first-child > td {\n  border-top: 0;\n}\n.table > tbody + tbody {\n  border-top: 2px solid #ddd;\n}\n.table .table {\n  background-color: #fff;\n}\n.table-condensed > thead > tr > th,\n.table-condensed > tbody > tr > th,\n.table-condensed > tfoot > tr > th,\n.table-condensed > thead > tr > td,\n.table-condensed > tbody > tr > td,\n.table-condensed > tfoot > tr > td {\n  padding: 2px;\n}\n.table-bordered {\n  border: 1px solid #ddd;\n}\n.table-bordered > thead > tr > th,\n.table-bordered > tbody > tr > th,\n.table-bordered > tfoot > tr > th,\n.table-bordered > thead > tr > td,\n.table-bordered > tbody > tr > td,\n.table-bordered > tfoot > tr > td {\n  border: 1px solid #ddd;\n}\n.table-bordered > thead > tr > th,\n.table-bordered > thead > tr > td {\n  border-bottom-width: 2px;\n}\n.table-striped > tbody > tr:nth-child(odd) > td,\n.table-striped > tbody > tr:nth-child(odd) > th {\n  background-color: #f9f9f9;\n}\n.table-hover > tbody > tr:hover > td,\n.table-hover > tbody > tr:hover > th {\n  background-color: #f5f5f5;\n}\ntable col[class*=\"col-\"] {\n  position: static;\n  display: table-column;\n  float: none;\n}\ntable td[class*=\"col-\"],\ntable th[class*=\"col-\"] {\n  position: static;\n  display: table-cell;\n  float: none;\n}\n.table > thead > tr > td.active,\n.table > tbody > tr > td.active,\n.table > tfoot > tr > td.active,\n.table > thead > tr > th.active,\n.table > tbody > tr > th.active,\n.table > tfoot > tr > th.active,\n.table > thead > tr.active > td,\n.table > tbody > tr.active > td,\n.table > tfoot > tr.active > td,\n.table > thead > tr.active > th,\n.table > tbody > tr.active > th,\n.table > tfoot > tr.active > th {\n  background-color: #f5f5f5;\n}\n.table-hover > tbody > tr > td.active:hover,\n.table-hover > tbody > tr > th.active:hover,\n.table-hover > tbody > tr.active:hover > td,\n.table-hover > tbody > tr.active:hover > th {\n  background-color: #e8e8e8;\n}\n.table > thead > tr > td.success,\n.table > tbody > tr > td.success,\n.table > tfoot > tr > td.success,\n.table > thead > tr > th.success,\n.table > tbody > tr > th.success,\n.table > tfoot > tr > th.success,\n.table > thead > tr.success > td,\n.table > tbody > tr.success > td,\n.table > tfoot > tr.success > td,\n.table > thead > tr.success > th,\n.table > tbody > tr.success > th,\n.table > tfoot > tr.success > th {\n  background-color: #dff0d8;\n}\n.table-hover > tbody > tr > td.success:hover,\n.table-hover > tbody > tr > th.success:hover,\n.table-hover > tbody > tr.success:hover > td,\n.table-hover > tbody > tr.success:hover > th {\n  background-color: #d0e9c6;\n}\n.table > thead > tr > td.info,\n.table > tbody > tr > td.info,\n.table > tfoot > tr > td.info,\n.table > thead > tr > th.info,\n.table > tbody > tr > th.info,\n.table > tfoot > tr > th.info,\n.table > thead > tr.info > td,\n.table > tbody > tr.info > td,\n.table > tfoot > tr.info > td,\n.table > thead > tr.info > th,\n.table > tbody > tr.info > th,\n.table > tfoot > tr.info > th {\n  background-color: #d9edf7;\n}\n.table-hover > tbody > tr > td.info:hover,\n.table-hover > tbody > tr > th.info:hover,\n.table-hover > tbody > tr.info:hover > td,\n.table-hover > tbody > tr.info:hover > th {\n  background-color: #c4e3f3;\n}\n.table > thead > tr > td.warning,\n.table > tbody > tr > td.warning,\n.table > tfoot > tr > td.warning,\n.table > thead > tr > th.warning,\n.table > tbody > tr > th.warning,\n.table > tfoot > tr > th.warning,\n.table > thead > tr.warning > td,\n.table > tbody > tr.warning > td,\n.table > tfoot > tr.warning > td,\n.table > thead > tr.warning > th,\n.table > tbody > tr.warning > th,\n.table > tfoot > tr.warning > th {\n  background-color: #fcf8e3;\n}\n.table-hover > tbody > tr > td.warning:hover,\n.table-hover > tbody > tr > th.warning:hover,\n.table-hover > tbody > tr.warning:hover > td,\n.table-hover > tbody > tr.warning:hover > th {\n  background-color: #faf2cc;\n}\n.table > thead > tr > td.danger,\n.table > tbody > tr > td.danger,\n.table > tfoot > tr > td.danger,\n.table > thead > tr > th.danger,\n.table > tbody > tr > th.danger,\n.table > tfoot > tr > th.danger,\n.table > thead > tr.danger > td,\n.table > tbody > tr.danger > td,\n.table > tfoot > tr.danger > td,\n.table > thead > tr.danger > th,\n.table > tbody > tr.danger > th,\n.table > tfoot > tr.danger > th {\n  background-color: #f2dede;\n}\n.table-hover > tbody > tr > td.danger:hover,\n.table-hover > tbody > tr > th.danger:hover,\n.table-hover > tbody > tr.danger:hover > td,\n.table-hover > tbody > tr.danger:hover > th {\n  background-color: #ebcccc;\n}\n@media (max-width: 767px) {\n  .table-responsive {\n    width: 100%;\n    margin-bottom: 15px;\n    overflow-x: scroll;\n    overflow-y: hidden;\n    -webkit-overflow-scrolling: touch;\n    -ms-overflow-style: -ms-autohiding-scrollbar;\n    border: 1px solid #ddd;\n  }\n  .table-responsive > .table {\n    margin-bottom: 0;\n  }\n  .table-responsive > .table > thead > tr > th,\n  .table-responsive > .table > tbody > tr > th,\n  .table-responsive > .table > tfoot > tr > th,\n  .table-responsive > .table > thead > tr > td,\n  .table-responsive > .table > tbody > tr > td,\n  .table-responsive > .table > tfoot > tr > td {\n    white-space: nowrap;\n  }\n  .table-responsive > .table-bordered {\n    border: 0;\n  }\n  .table-responsive > .table-bordered > thead > tr > th:first-child,\n  .table-responsive > .table-bordered > tbody > tr > th:first-child,\n  .table-responsive > .table-bordered > tfoot > tr > th:first-child,\n  .table-responsive > .table-bordered > thead > tr > td:first-child,\n  .table-responsive > .table-bordered > tbody > tr > td:first-child,\n  .table-responsive > .table-bordered > tfoot > tr > td:first-child {\n    border-left: 0;\n  }\n  .table-responsive > .table-bordered > thead > tr > th:last-child,\n  .table-responsive > .table-bordered > tbody > tr > th:last-child,\n  .table-responsive > .table-bordered > tfoot > tr > th:last-child,\n  .table-responsive > .table-bordered > thead > tr > td:last-child,\n  .table-responsive > .table-bordered > tbody > tr > td:last-child,\n  .table-responsive > .table-bordered > tfoot > tr > td:last-child {\n    border-right: 0;\n  }\n  .table-responsive > .table-bordered > tbody > tr:last-child > th,\n  .table-responsive > .table-bordered > tfoot > tr:last-child > th,\n  .table-responsive > .table-bordered > tbody > tr:last-child > td,\n  .table-responsive > .table-bordered > tfoot > tr:last-child > td {\n    border-bottom: 0;\n  }\n}\nfieldset {\n  min-width: 0;\n  padding: 0;\n  margin: 0;\n  border: 0;\n}\nlegend {\n  display: block;\n  width: 100%;\n  padding: 0;\n  margin-bottom: 20px;\n  font-size: 21px;\n  line-height: inherit;\n  color: #333;\n  border: 0;\n  border-bottom: 1px solid #e5e5e5;\n}\nlabel {\n  display: inline-block;\n  margin-bottom: 5px;\n  font-weight: bold;\n}\ninput[type=\"search\"] {\n  -webkit-box-sizing: border-box;\n     -moz-box-sizing: border-box;\n          box-sizing: border-box;\n}\ninput[type=\"radio\"],\ninput[type=\"checkbox\"] {\n  margin: 4px 0 0;\n  margin-top: 1px \\9;\n  /* IE8-9 */\n  line-height: normal;\n}\ninput[type=\"file\"] {\n  display: block;\n}\ninput[type=\"range\"] {\n  display: block;\n  width: 100%;\n}\nselect[multiple],\nselect[size] {\n  height: auto;\n}\ninput[type=\"file\"]:focus,\ninput[type=\"radio\"]:focus,\ninput[type=\"checkbox\"]:focus {\n  outline: thin dotted;\n  outline: 5px auto -webkit-focus-ring-color;\n  outline-offset: -2px;\n}\noutput {\n  display: block;\n  padding-top: 7px;\n  font-size: 14px;\n  line-height: 1.42857143;\n  color: #555;\n}\n.form-control {\n  display: block;\n  width: 100%;\n  height: 34px;\n  padding: 6px 12px;\n  font-size: 14px;\n  line-height: 1.42857143;\n  color: #555;\n  background-color: #fff;\n  background-image: none;\n  border: 1px solid #ccc;\n  border-radius: 4px;\n  -webkit-box-shadow: inset 0 1px 1px rgba(0, 0, 0, .075);\n          box-shadow: inset 0 1px 1px rgba(0, 0, 0, .075);\n  -webkit-transition: border-color ease-in-out .15s, box-shadow ease-in-out .15s;\n          transition: border-color ease-in-out .15s, box-shadow ease-in-out .15s;\n}\n.form-control:focus {\n  border-color: #66afe9;\n  outline: 0;\n  -webkit-box-shadow: inset 0 1px 1px rgba(0,0,0,.075), 0 0 8px rgba(102, 175, 233, .6);\n          box-shadow: inset 0 1px 1px rgba(0,0,0,.075), 0 0 8px rgba(102, 175, 233, .6);\n}\n.form-control::-moz-placeholder {\n  color: #999;\n  opacity: 1;\n}\n.form-control:-ms-input-placeholder {\n  color: #999;\n}\n.form-control::-webkit-input-placeholder {\n  color: #999;\n}\n.form-control[disabled],\n.form-control[readonly],\nfieldset[disabled] .form-control {\n  cursor: not-allowed;\n  background-color: #eee;\n  opacity: 1;\n}\ntextarea.form-control {\n  height: auto;\n}\ninput[type=\"search\"] {\n  -webkit-appearance: none;\n}\ninput[type=\"date\"] {\n  line-height: 34px;\n}\n.form-group {\n  margin-bottom: 15px;\n}\n.radio,\n.checkbox {\n  display: block;\n  min-height: 20px;\n  padding-left: 20px;\n  margin-top: 10px;\n  margin-bottom: 10px;\n}\n.radio label,\n.checkbox label {\n  display: inline;\n  font-weight: normal;\n  cursor: pointer;\n}\n.radio input[type=\"radio\"],\n.radio-inline input[type=\"radio\"],\n.checkbox input[type=\"checkbox\"],\n.checkbox-inline input[type=\"checkbox\"] {\n  float: left;\n  margin-left: -20px;\n}\n.radio + .radio,\n.checkbox + .checkbox {\n  margin-top: -5px;\n}\n.radio-inline,\n.checkbox-inline {\n  display: inline-block;\n  padding-left: 20px;\n  margin-bottom: 0;\n  font-weight: normal;\n  vertical-align: middle;\n  cursor: pointer;\n}\n.radio-inline + .radio-inline,\n.checkbox-inline + .checkbox-inline {\n  margin-top: 0;\n  margin-left: 10px;\n}\ninput[type=\"radio\"][disabled],\ninput[type=\"checkbox\"][disabled],\n.radio[disabled],\n.radio-inline[disabled],\n.checkbox[disabled],\n.checkbox-inline[disabled],\nfieldset[disabled] input[type=\"radio\"],\nfieldset[disabled] input[type=\"checkbox\"],\nfieldset[disabled] .radio,\nfieldset[disabled] .radio-inline,\nfieldset[disabled] .checkbox,\nfieldset[disabled] .checkbox-inline {\n  cursor: not-allowed;\n}\n.input-sm {\n  height: 30px;\n  padding: 5px 10px;\n  font-size: 12px;\n  line-height: 1.5;\n  border-radius: 3px;\n}\nselect.input-sm {\n  height: 30px;\n  line-height: 30px;\n}\ntextarea.input-sm,\nselect[multiple].input-sm {\n  height: auto;\n}\n.input-lg {\n  height: 46px;\n  padding: 10px 16px;\n  font-size: 18px;\n  line-height: 1.33;\n  border-radius: 6px;\n}\nselect.input-lg {\n  height: 46px;\n  line-height: 46px;\n}\ntextarea.input-lg,\nselect[multiple].input-lg {\n  height: auto;\n}\n.has-feedback {\n  position: relative;\n}\n.has-feedback .form-control {\n  padding-right: 42.5px;\n}\n.has-feedback .form-control-feedback {\n  position: absolute;\n  top: 25px;\n  right: 0;\n  display: block;\n  width: 34px;\n  height: 34px;\n  line-height: 34px;\n  text-align: center;\n}\n.has-success .help-block,\n.has-success .control-label,\n.has-success .radio,\n.has-success .checkbox,\n.has-success .radio-inline,\n.has-success .checkbox-inline {\n  color: #3c763d;\n}\n.has-success .form-control {\n  border-color: #3c763d;\n  -webkit-box-shadow: inset 0 1px 1px rgba(0, 0, 0, .075);\n          box-shadow: inset 0 1px 1px rgba(0, 0, 0, .075);\n}\n.has-success .form-control:focus {\n  border-color: #2b542c;\n  -webkit-box-shadow: inset 0 1px 1px rgba(0, 0, 0, .075), 0 0 6px #67b168;\n          box-shadow: inset 0 1px 1px rgba(0, 0, 0, .075), 0 0 6px #67b168;\n}\n.has-success .input-group-addon {\n  color: #3c763d;\n  background-color: #dff0d8;\n  border-color: #3c763d;\n}\n.has-success .form-control-feedback {\n  color: #3c763d;\n}\n.has-warning .help-block,\n.has-warning .control-label,\n.has-warning .radio,\n.has-warning .checkbox,\n.has-warning .radio-inline,\n.has-warning .checkbox-inline {\n  color: #8a6d3b;\n}\n.has-warning .form-control {\n  border-color: #8a6d3b;\n  -webkit-box-shadow: inset 0 1px 1px rgba(0, 0, 0, .075);\n          box-shadow: inset 0 1px 1px rgba(0, 0, 0, .075);\n}\n.has-warning .form-control:focus {\n  border-color: #66512c;\n  -webkit-box-shadow: inset 0 1px 1px rgba(0, 0, 0, .075), 0 0 6px #c0a16b;\n          box-shadow: inset 0 1px 1px rgba(0, 0, 0, .075), 0 0 6px #c0a16b;\n}\n.has-warning .input-group-addon {\n  color: #8a6d3b;\n  background-color: #fcf8e3;\n  border-color: #8a6d3b;\n}\n.has-warning .form-control-feedback {\n  color: #8a6d3b;\n}\n.has-error .help-block,\n.has-error .control-label,\n.has-error .radio,\n.has-error .checkbox,\n.has-error .radio-inline,\n.has-error .checkbox-inline {\n  color: #a94442;\n}\n.has-error .form-control {\n  border-color: #a94442;\n  -webkit-box-shadow: inset 0 1px 1px rgba(0, 0, 0, .075);\n          box-shadow: inset 0 1px 1px rgba(0, 0, 0, .075);\n}\n.has-error .form-control:focus {\n  border-color: #843534;\n  -webkit-box-shadow: inset 0 1px 1px rgba(0, 0, 0, .075), 0 0 6px #ce8483;\n          box-shadow: inset 0 1px 1px rgba(0, 0, 0, .075), 0 0 6px #ce8483;\n}\n.has-error .input-group-addon {\n  color: #a94442;\n  background-color: #f2dede;\n  border-color: #a94442;\n}\n.has-error .form-control-feedback {\n  color: #a94442;\n}\n.form-control-static {\n  margin-bottom: 0;\n}\n.help-block {\n  display: block;\n  margin-top: 5px;\n  margin-bottom: 10px;\n  color: #737373;\n}\n@media (min-width: 768px) {\n  .form-inline .form-group {\n    display: inline-block;\n    margin-bottom: 0;\n    vertical-align: middle;\n  }\n  .form-inline .form-control {\n    display: inline-block;\n    width: auto;\n    vertical-align: middle;\n  }\n  .form-inline .input-group > .form-control {\n    width: 100%;\n  }\n  .form-inline .control-label {\n    margin-bottom: 0;\n    vertical-align: middle;\n  }\n  .form-inline .radio,\n  .form-inline .checkbox {\n    display: inline-block;\n    padding-left: 0;\n    margin-top: 0;\n    margin-bottom: 0;\n    vertical-align: middle;\n  }\n  .form-inline .radio input[type=\"radio\"],\n  .form-inline .checkbox input[type=\"checkbox\"] {\n    float: none;\n    margin-left: 0;\n  }\n  .form-inline .has-feedback .form-control-feedback {\n    top: 0;\n  }\n}\n.form-horizontal .control-label,\n.form-horizontal .radio,\n.form-horizontal .checkbox,\n.form-horizontal .radio-inline,\n.form-horizontal .checkbox-inline {\n  padding-top: 7px;\n  margin-top: 0;\n  margin-bottom: 0;\n}\n.form-horizontal .radio,\n.form-horizontal .checkbox {\n  min-height: 27px;\n}\n.form-horizontal .form-group {\n  margin-right: -15px;\n  margin-left: -15px;\n}\n.form-horizontal .form-control-static {\n  padding-top: 7px;\n}\n@media (min-width: 768px) {\n  .form-horizontal .control-label {\n    text-align: right;\n  }\n}\n.form-horizontal .has-feedback .form-control-feedback {\n  top: 0;\n  right: 15px;\n}\n.btn {\n  display: inline-block;\n  padding: 6px 12px;\n  margin-bottom: 0;\n  font-size: 14px;\n  font-weight: normal;\n  line-height: 1.42857143;\n  text-align: center;\n  white-space: nowrap;\n  vertical-align: middle;\n  cursor: pointer;\n  -webkit-user-select: none;\n     -moz-user-select: none;\n      -ms-user-select: none;\n          user-select: none;\n  background-image: none;\n  border: 1px solid transparent;\n  border-radius: 4px;\n}\n.btn:focus,\n.btn:active:focus,\n.btn.active:focus {\n  outline: thin dotted;\n  outline: 5px auto -webkit-focus-ring-color;\n  outline-offset: -2px;\n}\n.btn:hover,\n.btn:focus {\n  color: #333;\n  text-decoration: none;\n}\n.btn:active,\n.btn.active {\n  background-image: none;\n  outline: 0;\n  -webkit-box-shadow: inset 0 3px 5px rgba(0, 0, 0, .125);\n          box-shadow: inset 0 3px 5px rgba(0, 0, 0, .125);\n}\n.btn.disabled,\n.btn[disabled],\nfieldset[disabled] .btn {\n  pointer-events: none;\n  cursor: not-allowed;\n  filter: alpha(opacity=65);\n  -webkit-box-shadow: none;\n          box-shadow: none;\n  opacity: .65;\n}\n.btn-default {\n  color: #333;\n  background-color: #fff;\n  border-color: #ccc;\n}\n.btn-default:hover,\n.btn-default:focus,\n.btn-default:active,\n.btn-default.active,\n.open .dropdown-toggle.btn-default {\n  color: #333;\n  background-color: #ebebeb;\n  border-color: #adadad;\n}\n.btn-default:active,\n.btn-default.active,\n.open .dropdown-toggle.btn-default {\n  background-image: none;\n}\n.btn-default.disabled,\n.btn-default[disabled],\nfieldset[disabled] .btn-default,\n.btn-default.disabled:hover,\n.btn-default[disabled]:hover,\nfieldset[disabled] .btn-default:hover,\n.btn-default.disabled:focus,\n.btn-default[disabled]:focus,\nfieldset[disabled] .btn-default:focus,\n.btn-default.disabled:active,\n.btn-default[disabled]:active,\nfieldset[disabled] .btn-default:active,\n.btn-default.disabled.active,\n.btn-default[disabled].active,\nfieldset[disabled] .btn-default.active {\n  background-color: #fff;\n  border-color: #ccc;\n}\n.btn-default .badge {\n  color: #fff;\n  background-color: #333;\n}\n.btn-primary {\n  color: #fff;\n  background-color: #428bca;\n  border-color: #357ebd;\n}\n.btn-primary:hover,\n.btn-primary:focus,\n.btn-primary:active,\n.btn-primary.active,\n.open .dropdown-toggle.btn-primary {\n  color: #fff;\n  background-color: #3276b1;\n  border-color: #285e8e;\n}\n.btn-primary:active,\n.btn-primary.active,\n.open .dropdown-toggle.btn-primary {\n  background-image: none;\n}\n.btn-primary.disabled,\n.btn-primary[disabled],\nfieldset[disabled] .btn-primary,\n.btn-primary.disabled:hover,\n.btn-primary[disabled]:hover,\nfieldset[disabled] .btn-primary:hover,\n.btn-primary.disabled:focus,\n.btn-primary[disabled]:focus,\nfieldset[disabled] .btn-primary:focus,\n.btn-primary.disabled:active,\n.btn-primary[disabled]:active,\nfieldset[disabled] .btn-primary:active,\n.btn-primary.disabled.active,\n.btn-primary[disabled].active,\nfieldset[disabled] .btn-primary.active {\n  background-color: #428bca;\n  border-color: #357ebd;\n}\n.btn-primary .badge {\n  color: #428bca;\n  background-color: #fff;\n}\n.btn-success {\n  color: #fff;\n  background-color: #5cb85c;\n  border-color: #4cae4c;\n}\n.btn-success:hover,\n.btn-success:focus,\n.btn-success:active,\n.btn-success.active,\n.open .dropdown-toggle.btn-success {\n  color: #fff;\n  background-color: #47a447;\n  border-color: #398439;\n}\n.btn-success:active,\n.btn-success.active,\n.open .dropdown-toggle.btn-success {\n  background-image: none;\n}\n.btn-success.disabled,\n.btn-success[disabled],\nfieldset[disabled] .btn-success,\n.btn-success.disabled:hover,\n.btn-success[disabled]:hover,\nfieldset[disabled] .btn-success:hover,\n.btn-success.disabled:focus,\n.btn-success[disabled]:focus,\nfieldset[disabled] .btn-success:focus,\n.btn-success.disabled:active,\n.btn-success[disabled]:active,\nfieldset[disabled] .btn-success:active,\n.btn-success.disabled.active,\n.btn-success[disabled].active,\nfieldset[disabled] .btn-success.active {\n  background-color: #5cb85c;\n  border-color: #4cae4c;\n}\n.btn-success .badge {\n  color: #5cb85c;\n  background-color: #fff;\n}\n.btn-info {\n  color: #fff;\n  background-color: #5bc0de;\n  border-color: #46b8da;\n}\n.btn-info:hover,\n.btn-info:focus,\n.btn-info:active,\n.btn-info.active,\n.open .dropdown-toggle.btn-info {\n  color: #fff;\n  background-color: #39b3d7;\n  border-color: #269abc;\n}\n.btn-info:active,\n.btn-info.active,\n.open .dropdown-toggle.btn-info {\n  background-image: none;\n}\n.btn-info.disabled,\n.btn-info[disabled],\nfieldset[disabled] .btn-info,\n.btn-info.disabled:hover,\n.btn-info[disabled]:hover,\nfieldset[disabled] .btn-info:hover,\n.btn-info.disabled:focus,\n.btn-info[disabled]:focus,\nfieldset[disabled] .btn-info:focus,\n.btn-info.disabled:active,\n.btn-info[disabled]:active,\nfieldset[disabled] .btn-info:active,\n.btn-info.disabled.active,\n.btn-info[disabled].active,\nfieldset[disabled] .btn-info.active {\n  background-color: #5bc0de;\n  border-color: #46b8da;\n}\n.btn-info .badge {\n  color: #5bc0de;\n  background-color: #fff;\n}\n.btn-warning {\n  color: #fff;\n  background-color: #f0ad4e;\n  border-color: #eea236;\n}\n.btn-warning:hover,\n.btn-warning:focus,\n.btn-warning:active,\n.btn-warning.active,\n.open .dropdown-toggle.btn-warning {\n  color: #fff;\n  background-color: #ed9c28;\n  border-color: #d58512;\n}\n.btn-warning:active,\n.btn-warning.active,\n.open .dropdown-toggle.btn-warning {\n  background-image: none;\n}\n.btn-warning.disabled,\n.btn-warning[disabled],\nfieldset[disabled] .btn-warning,\n.btn-warning.disabled:hover,\n.btn-warning[disabled]:hover,\nfieldset[disabled] .btn-warning:hover,\n.btn-warning.disabled:focus,\n.btn-warning[disabled]:focus,\nfieldset[disabled] .btn-warning:focus,\n.btn-warning.disabled:active,\n.btn-warning[disabled]:active,\nfieldset[disabled] .btn-warning:active,\n.btn-warning.disabled.active,\n.btn-warning[disabled].active,\nfieldset[disabled] .btn-warning.active {\n  background-color: #f0ad4e;\n  border-color: #eea236;\n}\n.btn-warning .badge {\n  color: #f0ad4e;\n  background-color: #fff;\n}\n.btn-danger {\n  color: #fff;\n  background-color: #d9534f;\n  border-color: #d43f3a;\n}\n.btn-danger:hover,\n.btn-danger:focus,\n.btn-danger:active,\n.btn-danger.active,\n.open .dropdown-toggle.btn-danger {\n  color: #fff;\n  background-color: #d2322d;\n  border-color: #ac2925;\n}\n.btn-danger:active,\n.btn-danger.active,\n.open .dropdown-toggle.btn-danger {\n  background-image: none;\n}\n.btn-danger.disabled,\n.btn-danger[disabled],\nfieldset[disabled] .btn-danger,\n.btn-danger.disabled:hover,\n.btn-danger[disabled]:hover,\nfieldset[disabled] .btn-danger:hover,\n.btn-danger.disabled:focus,\n.btn-danger[disabled]:focus,\nfieldset[disabled] .btn-danger:focus,\n.btn-danger.disabled:active,\n.btn-danger[disabled]:active,\nfieldset[disabled] .btn-danger:active,\n.btn-danger.disabled.active,\n.btn-danger[disabled].active,\nfieldset[disabled] .btn-danger.active {\n  background-color: #d9534f;\n  border-color: #d43f3a;\n}\n.btn-danger .badge {\n  color: #d9534f;\n  background-color: #fff;\n}\n.btn-link {\n  font-weight: normal;\n  color: #428bca;\n  cursor: pointer;\n  border-radius: 0;\n}\n.btn-link,\n.btn-link:active,\n.btn-link[disabled],\nfieldset[disabled] .btn-link {\n  background-color: transparent;\n  -webkit-box-shadow: none;\n          box-shadow: none;\n}\n.btn-link,\n.btn-link:hover,\n.btn-link:focus,\n.btn-link:active {\n  border-color: transparent;\n}\n.btn-link:hover,\n.btn-link:focus {\n  color: #2a6496;\n  text-decoration: underline;\n  background-color: transparent;\n}\n.btn-link[disabled]:hover,\nfieldset[disabled] .btn-link:hover,\n.btn-link[disabled]:focus,\nfieldset[disabled] .btn-link:focus {\n  color: #999;\n  text-decoration: none;\n}\n.btn-lg,\n.btn-group-lg > .btn {\n  padding: 10px 16px;\n  font-size: 18px;\n  line-height: 1.33;\n  border-radius: 6px;\n}\n.btn-sm,\n.btn-group-sm > .btn {\n  padding: 5px 10px;\n  font-size: 12px;\n  line-height: 1.5;\n  border-radius: 3px;\n}\n.btn-xs,\n.btn-group-xs > .btn {\n  padding: 1px 5px;\n  font-size: 12px;\n  line-height: 1.5;\n  border-radius: 3px;\n}\n.btn-block {\n  display: block;\n  width: 100%;\n  padding-right: 0;\n  padding-left: 0;\n}\n.btn-block + .btn-block {\n  margin-top: 5px;\n}\ninput[type=\"submit\"].btn-block,\ninput[type=\"reset\"].btn-block,\ninput[type=\"button\"].btn-block {\n  width: 100%;\n}\n.fade {\n  opacity: 0;\n  -webkit-transition: opacity .15s linear;\n          transition: opacity .15s linear;\n}\n.fade.in {\n  opacity: 1;\n}\n.collapse {\n  display: none;\n}\n.collapse.in {\n  display: block;\n}\n.collapsing {\n  position: relative;\n  height: 0;\n  overflow: hidden;\n  -webkit-transition: height .35s ease;\n          transition: height .35s ease;\n}\n@font-face {\n  font-family: 'Glyphicons Halflings';\n\n  src: url('../fonts/glyphicons-halflings-regular.eot');\n  src: url('../fonts/glyphicons-halflings-regular.eot?#iefix') format('embedded-opentype'), url('../fonts/glyphicons-halflings-regular.woff') format('woff'), url('../fonts/glyphicons-halflings-regular.ttf') format('truetype'), url('../fonts/glyphicons-halflings-regular.svg#glyphicons_halflingsregular') format('svg');\n}\n.glyphicon {\n  position: relative;\n  top: 1px;\n  display: inline-block;\n  font-family: 'Glyphicons Halflings';\n  font-style: normal;\n  font-weight: normal;\n  line-height: 1;\n\n  -webkit-font-smoothing: antialiased;\n  -moz-osx-font-smoothing: grayscale;\n}\n.glyphicon-asterisk:before {\n  content: \"\\2a\";\n}\n.glyphicon-plus:before {\n  content: \"\\2b\";\n}\n.glyphicon-euro:before {\n  content: \"\\20ac\";\n}\n.glyphicon-minus:before {\n  content: \"\\2212\";\n}\n.glyphicon-cloud:before {\n  content: \"\\2601\";\n}\n.glyphicon-envelope:before {\n  content: \"\\2709\";\n}\n.glyphicon-pencil:before {\n  content: \"\\270f\";\n}\n.glyphicon-glass:before {\n  content: \"\\e001\";\n}\n.glyphicon-music:before {\n  content: \"\\e002\";\n}\n.glyphicon-search:before {\n  content: \"\\e003\";\n}\n.glyphicon-heart:before {\n  content: \"\\e005\";\n}\n.glyphicon-star:before {\n  content: \"\\e006\";\n}\n.glyphicon-star-empty:before {\n  content: \"\\e007\";\n}\n.glyphicon-user:before {\n  content: \"\\e008\";\n}\n.glyphicon-film:before {\n  content: \"\\e009\";\n}\n.glyphicon-th-large:before {\n  content: \"\\e010\";\n}\n.glyphicon-th:before {\n  content: \"\\e011\";\n}\n.glyphicon-th-list:before {\n  content: \"\\e012\";\n}\n.glyphicon-ok:before {\n  content: \"\\e013\";\n}\n.glyphicon-remove:before {\n  content: \"\\e014\";\n}\n.glyphicon-zoom-in:before {\n  content: \"\\e015\";\n}\n.glyphicon-zoom-out:before {\n  content: \"\\e016\";\n}\n.glyphicon-off:before {\n  content: \"\\e017\";\n}\n.glyphicon-signal:before {\n  content: \"\\e018\";\n}\n.glyphicon-cog:before {\n  content: \"\\e019\";\n}\n.glyphicon-trash:before {\n  content: \"\\e020\";\n}\n.glyphicon-home:before {\n  content: \"\\e021\";\n}\n.glyphicon-file:before {\n  content: \"\\e022\";\n}\n.glyphicon-time:before {\n  content: \"\\e023\";\n}\n.glyphicon-road:before {\n  content: \"\\e024\";\n}\n.glyphicon-download-alt:before {\n  content: \"\\e025\";\n}\n.glyphicon-download:before {\n  content: \"\\e026\";\n}\n.glyphicon-upload:before {\n  content: \"\\e027\";\n}\n.glyphicon-inbox:before {\n  content: \"\\e028\";\n}\n.glyphicon-play-circle:before {\n  content: \"\\e029\";\n}\n.glyphicon-repeat:before {\n  content: \"\\e030\";\n}\n.glyphicon-refresh:before {\n  content: \"\\e031\";\n}\n.glyphicon-list-alt:before {\n  content: \"\\e032\";\n}\n.glyphicon-lock:before {\n  content: \"\\e033\";\n}\n.glyphicon-flag:before {\n  content: \"\\e034\";\n}\n.glyphicon-headphones:before {\n  content: \"\\e035\";\n}\n.glyphicon-volume-off:before {\n  content: \"\\e036\";\n}\n.glyphicon-volume-down:before {\n  content: \"\\e037\";\n}\n.glyphicon-volume-up:before {\n  content: \"\\e038\";\n}\n.glyphicon-qrcode:before {\n  content: \"\\e039\";\n}\n.glyphicon-barcode:before {\n  content: \"\\e040\";\n}\n.glyphicon-tag:before {\n  content: \"\\e041\";\n}\n.glyphicon-tags:before {\n  content: \"\\e042\";\n}\n.glyphicon-book:before {\n  content: \"\\e043\";\n}\n.glyphicon-bookmark:before {\n  content: \"\\e044\";\n}\n.glyphicon-print:before {\n  content: \"\\e045\";\n}\n.glyphicon-camera:before {\n  content: \"\\e046\";\n}\n.glyphicon-font:before {\n  content: \"\\e047\";\n}\n.glyphicon-bold:before {\n  content: \"\\e048\";\n}\n.glyphicon-italic:before {\n  content: \"\\e049\";\n}\n.glyphicon-text-height:before {\n  content: \"\\e050\";\n}\n.glyphicon-text-width:before {\n  content: \"\\e051\";\n}\n.glyphicon-align-left:before {\n  content: \"\\e052\";\n}\n.glyphicon-align-center:before {\n  content: \"\\e053\";\n}\n.glyphicon-align-right:before {\n  content: \"\\e054\";\n}\n.glyphicon-align-justify:before {\n  content: \"\\e055\";\n}\n.glyphicon-list:before {\n  content: \"\\e056\";\n}\n.glyphicon-indent-left:before {\n  content: \"\\e057\";\n}\n.glyphicon-indent-right:before {\n  content: \"\\e058\";\n}\n.glyphicon-facetime-video:before {\n  content: \"\\e059\";\n}\n.glyphicon-picture:before {\n  content: \"\\e060\";\n}\n.glyphicon-map-marker:before {\n  content: \"\\e062\";\n}\n.glyphicon-adjust:before {\n  content: \"\\e063\";\n}\n.glyphicon-tint:before {\n  content: \"\\e064\";\n}\n.glyphicon-edit:before {\n  content: \"\\e065\";\n}\n.glyphicon-share:before {\n  content: \"\\e066\";\n}\n.glyphicon-check:before {\n  content: \"\\e067\";\n}\n.glyphicon-move:before {\n  content: \"\\e068\";\n}\n.glyphicon-step-backward:before {\n  content: \"\\e069\";\n}\n.glyphicon-fast-backward:before {\n  content: \"\\e070\";\n}\n.glyphicon-backward:before {\n  content: \"\\e071\";\n}\n.glyphicon-play:before {\n  content: \"\\e072\";\n}\n.glyphicon-pause:before {\n  content: \"\\e073\";\n}\n.glyphicon-stop:before {\n  content: \"\\e074\";\n}\n.glyphicon-forward:before {\n  content: \"\\e075\";\n}\n.glyphicon-fast-forward:before {\n  content: \"\\e076\";\n}\n.glyphicon-step-forward:before {\n  content: \"\\e077\";\n}\n.glyphicon-eject:before {\n  content: \"\\e078\";\n}\n.glyphicon-chevron-left:before {\n  content: \"\\e079\";\n}\n.glyphicon-chevron-right:before {\n  content: \"\\e080\";\n}\n.glyphicon-plus-sign:before {\n  content: \"\\e081\";\n}\n.glyphicon-minus-sign:before {\n  content: \"\\e082\";\n}\n.glyphicon-remove-sign:before {\n  content: \"\\e083\";\n}\n.glyphicon-ok-sign:before {\n  content: \"\\e084\";\n}\n.glyphicon-question-sign:before {\n  content: \"\\e085\";\n}\n.glyphicon-info-sign:before {\n  content: \"\\e086\";\n}\n.glyphicon-screenshot:before {\n  content: \"\\e087\";\n}\n.glyphicon-remove-circle:before {\n  content: \"\\e088\";\n}\n.glyphicon-ok-circle:before {\n  content: \"\\e089\";\n}\n.glyphicon-ban-circle:before {\n  content: \"\\e090\";\n}\n.glyphicon-arrow-left:before {\n  content: \"\\e091\";\n}\n.glyphicon-arrow-right:before {\n  content: \"\\e092\";\n}\n.glyphicon-arrow-up:before {\n  content: \"\\e093\";\n}\n.glyphicon-arrow-down:before {\n  content: \"\\e094\";\n}\n.glyphicon-share-alt:before {\n  content: \"\\e095\";\n}\n.glyphicon-resize-full:before {\n  content: \"\\e096\";\n}\n.glyphicon-resize-small:before {\n  content: \"\\e097\";\n}\n.glyphicon-exclamation-sign:before {\n  content: \"\\e101\";\n}\n.glyphicon-gift:before {\n  content: \"\\e102\";\n}\n.glyphicon-leaf:before {\n  content: \"\\e103\";\n}\n.glyphicon-fire:before {\n  content: \"\\e104\";\n}\n.glyphicon-eye-open:before {\n  content: \"\\e105\";\n}\n.glyphicon-eye-close:before {\n  content: \"\\e106\";\n}\n.glyphicon-warning-sign:before {\n  content: \"\\e107\";\n}\n.glyphicon-plane:before {\n  content: \"\\e108\";\n}\n.glyphicon-calendar:before {\n  content: \"\\e109\";\n}\n.glyphicon-random:before {\n  content: \"\\e110\";\n}\n.glyphicon-comment:before {\n  content: \"\\e111\";\n}\n.glyphicon-magnet:before {\n  content: \"\\e112\";\n}\n.glyphicon-chevron-up:before {\n  content: \"\\e113\";\n}\n.glyphicon-chevron-down:before {\n  content: \"\\e114\";\n}\n.glyphicon-retweet:before {\n  content: \"\\e115\";\n}\n.glyphicon-shopping-cart:before {\n  content: \"\\e116\";\n}\n.glyphicon-folder-close:before {\n  content: \"\\e117\";\n}\n.glyphicon-folder-open:before {\n  content: \"\\e118\";\n}\n.glyphicon-resize-vertical:before {\n  content: \"\\e119\";\n}\n.glyphicon-resize-horizontal:before {\n  content: \"\\e120\";\n}\n.glyphicon-hdd:before {\n  content: \"\\e121\";\n}\n.glyphicon-bullhorn:before {\n  content: \"\\e122\";\n}\n.glyphicon-bell:before {\n  content: \"\\e123\";\n}\n.glyphicon-certificate:before {\n  content: \"\\e124\";\n}\n.glyphicon-thumbs-up:before {\n  content: \"\\e125\";\n}\n.glyphicon-thumbs-down:before {\n  content: \"\\e126\";\n}\n.glyphicon-hand-right:before {\n  content: \"\\e127\";\n}\n.glyphicon-hand-left:before {\n  content: \"\\e128\";\n}\n.glyphicon-hand-up:before {\n  content: \"\\e129\";\n}\n.glyphicon-hand-down:before {\n  content: \"\\e130\";\n}\n.glyphicon-circle-arrow-right:before {\n  content: \"\\e131\";\n}\n.glyphicon-circle-arrow-left:before {\n  content: \"\\e132\";\n}\n.glyphicon-circle-arrow-up:before {\n  content: \"\\e133\";\n}\n.glyphicon-circle-arrow-down:before {\n  content: \"\\e134\";\n}\n.glyphicon-globe:before {\n  content: \"\\e135\";\n}\n.glyphicon-wrench:before {\n  content: \"\\e136\";\n}\n.glyphicon-tasks:before {\n  content: \"\\e137\";\n}\n.glyphicon-filter:before {\n  content: \"\\e138\";\n}\n.glyphicon-briefcase:before {\n  content: \"\\e139\";\n}\n.glyphicon-fullscreen:before {\n  content: \"\\e140\";\n}\n.glyphicon-dashboard:before {\n  content: \"\\e141\";\n}\n.glyphicon-paperclip:before {\n  content: \"\\e142\";\n}\n.glyphicon-heart-empty:before {\n  content: \"\\e143\";\n}\n.glyphicon-link:before {\n  content: \"\\e144\";\n}\n.glyphicon-phone:before {\n  content: \"\\e145\";\n}\n.glyphicon-pushpin:before {\n  content: \"\\e146\";\n}\n.glyphicon-usd:before {\n  content: \"\\e148\";\n}\n.glyphicon-gbp:before {\n  content: \"\\e149\";\n}\n.glyphicon-sort:before {\n  content: \"\\e150\";\n}\n.glyphicon-sort-by-alphabet:before {\n  content: \"\\e151\";\n}\n.glyphicon-sort-by-alphabet-alt:before {\n  content: \"\\e152\";\n}\n.glyphicon-sort-by-order:before {\n  content: \"\\e153\";\n}\n.glyphicon-sort-by-order-alt:before {\n  content: \"\\e154\";\n}\n.glyphicon-sort-by-attributes:before {\n  content: \"\\e155\";\n}\n.glyphicon-sort-by-attributes-alt:before {\n  content: \"\\e156\";\n}\n.glyphicon-unchecked:before {\n  content: \"\\e157\";\n}\n.glyphicon-expand:before {\n  content: \"\\e158\";\n}\n.glyphicon-collapse-down:before {\n  content: \"\\e159\";\n}\n.glyphicon-collapse-up:before {\n  content: \"\\e160\";\n}\n.glyphicon-log-in:before {\n  content: \"\\e161\";\n}\n.glyphicon-flash:before {\n  content: \"\\e162\";\n}\n.glyphicon-log-out:before {\n  content: \"\\e163\";\n}\n.glyphicon-new-window:before {\n  content: \"\\e164\";\n}\n.glyphicon-record:before {\n  content: \"\\e165\";\n}\n.glyphicon-save:before {\n  content: \"\\e166\";\n}\n.glyphicon-open:before {\n  content: \"\\e167\";\n}\n.glyphicon-saved:before {\n  content: \"\\e168\";\n}\n.glyphicon-import:before {\n  content: \"\\e169\";\n}\n.glyphicon-export:before {\n  content: \"\\e170\";\n}\n.glyphicon-send:before {\n  content: \"\\e171\";\n}\n.glyphicon-floppy-disk:before {\n  content: \"\\e172\";\n}\n.glyphicon-floppy-saved:before {\n  content: \"\\e173\";\n}\n.glyphicon-floppy-remove:before {\n  content: \"\\e174\";\n}\n.glyphicon-floppy-save:before {\n  content: \"\\e175\";\n}\n.glyphicon-floppy-open:before {\n  content: \"\\e176\";\n}\n.glyphicon-credit-card:before {\n  content: \"\\e177\";\n}\n.glyphicon-transfer:before {\n  content: \"\\e178\";\n}\n.glyphicon-cutlery:before {\n  content: \"\\e179\";\n}\n.glyphicon-header:before {\n  content: \"\\e180\";\n}\n.glyphicon-compressed:before {\n  content: \"\\e181\";\n}\n.glyphicon-earphone:before {\n  content: \"\\e182\";\n}\n.glyphicon-phone-alt:before {\n  content: \"\\e183\";\n}\n.glyphicon-tower:before {\n  content: \"\\e184\";\n}\n.glyphicon-stats:before {\n  content: \"\\e185\";\n}\n.glyphicon-sd-video:before {\n  content: \"\\e186\";\n}\n.glyphicon-hd-video:before {\n  content: \"\\e187\";\n}\n.glyphicon-subtitles:before {\n  content: \"\\e188\";\n}\n.glyphicon-sound-stereo:before {\n  content: \"\\e189\";\n}\n.glyphicon-sound-dolby:before {\n  content: \"\\e190\";\n}\n.glyphicon-sound-5-1:before {\n  content: \"\\e191\";\n}\n.glyphicon-sound-6-1:before {\n  content: \"\\e192\";\n}\n.glyphicon-sound-7-1:before {\n  content: \"\\e193\";\n}\n.glyphicon-copyright-mark:before {\n  content: \"\\e194\";\n}\n.glyphicon-registration-mark:before {\n  content: \"\\e195\";\n}\n.glyphicon-cloud-download:before {\n  content: \"\\e197\";\n}\n.glyphicon-cloud-upload:before {\n  content: \"\\e198\";\n}\n.glyphicon-tree-conifer:before {\n  content: \"\\e199\";\n}\n.glyphicon-tree-deciduous:before {\n  content: \"\\e200\";\n}\n.caret {\n  display: inline-block;\n  width: 0;\n  height: 0;\n  margin-left: 2px;\n  vertical-align: middle;\n  border-top: 4px solid;\n  border-right: 4px solid transparent;\n  border-left: 4px solid transparent;\n}\n.dropdown {\n  position: relative;\n}\n.dropdown-toggle:focus {\n  outline: 0;\n}\n.dropdown-menu {\n  position: absolute;\n  top: 100%;\n  left: 0;\n  z-index: 1000;\n  display: none;\n  float: left;\n  min-width: 160px;\n  padding: 5px 0;\n  margin: 2px 0 0;\n  font-size: 14px;\n  list-style: none;\n  background-color: #fff;\n  background-clip: padding-box;\n  border: 1px solid #ccc;\n  border: 1px solid rgba(0, 0, 0, .15);\n  border-radius: 4px;\n  -webkit-box-shadow: 0 6px 12px rgba(0, 0, 0, .175);\n          box-shadow: 0 6px 12px rgba(0, 0, 0, .175);\n}\n.dropdown-menu.pull-right {\n  right: 0;\n  left: auto;\n}\n.dropdown-menu .divider {\n  height: 1px;\n  margin: 9px 0;\n  overflow: hidden;\n  background-color: #e5e5e5;\n}\n.dropdown-menu > li > a {\n  display: block;\n  padding: 3px 20px;\n  clear: both;\n  font-weight: normal;\n  line-height: 1.42857143;\n  color: #333;\n  white-space: nowrap;\n}\n.dropdown-menu > li > a:hover,\n.dropdown-menu > li > a:focus {\n  color: #262626;\n  text-decoration: none;\n  background-color: #f5f5f5;\n}\n.dropdown-menu > .active > a,\n.dropdown-menu > .active > a:hover,\n.dropdown-menu > .active > a:focus {\n  color: #fff;\n  text-decoration: none;\n  background-color: #428bca;\n  outline: 0;\n}\n.dropdown-menu > .disabled > a,\n.dropdown-menu > .disabled > a:hover,\n.dropdown-menu > .disabled > a:focus {\n  color: #999;\n}\n.dropdown-menu > .disabled > a:hover,\n.dropdown-menu > .disabled > a:focus {\n  text-decoration: none;\n  cursor: not-allowed;\n  background-color: transparent;\n  background-image: none;\n  filter: progid:DXImageTransform.Microsoft.gradient(enabled = false);\n}\n.open > .dropdown-menu {\n  display: block;\n}\n.open > a {\n  outline: 0;\n}\n.dropdown-menu-right {\n  right: 0;\n  left: auto;\n}\n.dropdown-menu-left {\n  right: auto;\n  left: 0;\n}\n.dropdown-header {\n  display: block;\n  padding: 3px 20px;\n  font-size: 12px;\n  line-height: 1.42857143;\n  color: #999;\n}\n.dropdown-backdrop {\n  position: fixed;\n  top: 0;\n  right: 0;\n  bottom: 0;\n  left: 0;\n  z-index: 990;\n}\n.pull-right > .dropdown-menu {\n  right: 0;\n  left: auto;\n}\n.dropup .caret,\n.navbar-fixed-bottom .dropdown .caret {\n  content: \"\";\n  border-top: 0;\n  border-bottom: 4px solid;\n}\n.dropup .dropdown-menu,\n.navbar-fixed-bottom .dropdown .dropdown-menu {\n  top: auto;\n  bottom: 100%;\n  margin-bottom: 1px;\n}\n@media (min-width: 768px) {\n  .navbar-right .dropdown-menu {\n    right: 0;\n    left: auto;\n  }\n  .navbar-right .dropdown-menu-left {\n    right: auto;\n    left: 0;\n  }\n}\n.btn-group,\n.btn-group-vertical {\n  position: relative;\n  display: inline-block;\n  vertical-align: middle;\n}\n.btn-group > .btn,\n.btn-group-vertical > .btn {\n  position: relative;\n  float: left;\n}\n.btn-group > .btn:hover,\n.btn-group-vertical > .btn:hover,\n.btn-group > .btn:focus,\n.btn-group-vertical > .btn:focus,\n.btn-group > .btn:active,\n.btn-group-vertical > .btn:active,\n.btn-group > .btn.active,\n.btn-group-vertical > .btn.active {\n  z-index: 2;\n}\n.btn-group > .btn:focus,\n.btn-group-vertical > .btn:focus {\n  outline: none;\n}\n.btn-group .btn + .btn,\n.btn-group .btn + .btn-group,\n.btn-group .btn-group + .btn,\n.btn-group .btn-group + .btn-group {\n  margin-left: -1px;\n}\n.btn-toolbar {\n  margin-left: -5px;\n}\n.btn-toolbar .btn-group,\n.btn-toolbar .input-group {\n  float: left;\n}\n.btn-toolbar > .btn,\n.btn-toolbar > .btn-group,\n.btn-toolbar > .input-group {\n  margin-left: 5px;\n}\n.btn-group > .btn:not(:first-child):not(:last-child):not(.dropdown-toggle) {\n  border-radius: 0;\n}\n.btn-group > .btn:first-child {\n  margin-left: 0;\n}\n.btn-group > .btn:first-child:not(:last-child):not(.dropdown-toggle) {\n  border-top-right-radius: 0;\n  border-bottom-right-radius: 0;\n}\n.btn-group > .btn:last-child:not(:first-child),\n.btn-group > .dropdown-toggle:not(:first-child) {\n  border-top-left-radius: 0;\n  border-bottom-left-radius: 0;\n}\n.btn-group > .btn-group {\n  float: left;\n}\n.btn-group > .btn-group:not(:first-child):not(:last-child) > .btn {\n  border-radius: 0;\n}\n.btn-group > .btn-group:first-child > .btn:last-child,\n.btn-group > .btn-group:first-child > .dropdown-toggle {\n  border-top-right-radius: 0;\n  border-bottom-right-radius: 0;\n}\n.btn-group > .btn-group:last-child > .btn:first-child {\n  border-top-left-radius: 0;\n  border-bottom-left-radius: 0;\n}\n.btn-group .dropdown-toggle:active,\n.btn-group.open .dropdown-toggle {\n  outline: 0;\n}\n.btn-group > .btn + .dropdown-toggle {\n  padding-right: 8px;\n  padding-left: 8px;\n}\n.btn-group > .btn-lg + .dropdown-toggle {\n  padding-right: 12px;\n  padding-left: 12px;\n}\n.btn-group.open .dropdown-toggle {\n  -webkit-box-shadow: inset 0 3px 5px rgba(0, 0, 0, .125);\n          box-shadow: inset 0 3px 5px rgba(0, 0, 0, .125);\n}\n.btn-group.open .dropdown-toggle.btn-link {\n  -webkit-box-shadow: none;\n          box-shadow: none;\n}\n.btn .caret {\n  margin-left: 0;\n}\n.btn-lg .caret {\n  border-width: 5px 5px 0;\n  border-bottom-width: 0;\n}\n.dropup .btn-lg .caret {\n  border-width: 0 5px 5px;\n}\n.btn-group-vertical > .btn,\n.btn-group-vertical > .btn-group,\n.btn-group-vertical > .btn-group > .btn {\n  display: block;\n  float: none;\n  width: 100%;\n  max-width: 100%;\n}\n.btn-group-vertical > .btn-group > .btn {\n  float: none;\n}\n.btn-group-vertical > .btn + .btn,\n.btn-group-vertical > .btn + .btn-group,\n.btn-group-vertical > .btn-group + .btn,\n.btn-group-vertical > .btn-group + .btn-group {\n  margin-top: -1px;\n  margin-left: 0;\n}\n.btn-group-vertical > .btn:not(:first-child):not(:last-child) {\n  border-radius: 0;\n}\n.btn-group-vertical > .btn:first-child:not(:last-child) {\n  border-top-right-radius: 4px;\n  border-bottom-right-radius: 0;\n  border-bottom-left-radius: 0;\n}\n.btn-group-vertical > .btn:last-child:not(:first-child) {\n  border-top-left-radius: 0;\n  border-top-right-radius: 0;\n  border-bottom-left-radius: 4px;\n}\n.btn-group-vertical > .btn-group:not(:first-child):not(:last-child) > .btn {\n  border-radius: 0;\n}\n.btn-group-vertical > .btn-group:first-child:not(:last-child) > .btn:last-child,\n.btn-group-vertical > .btn-group:first-child:not(:last-child) > .dropdown-toggle {\n  border-bottom-right-radius: 0;\n  border-bottom-left-radius: 0;\n}\n.btn-group-vertical > .btn-group:last-child:not(:first-child) > .btn:first-child {\n  border-top-left-radius: 0;\n  border-top-right-radius: 0;\n}\n.btn-group-justified {\n  display: table;\n  width: 100%;\n  table-layout: fixed;\n  border-collapse: separate;\n}\n.btn-group-justified > .btn,\n.btn-group-justified > .btn-group {\n  display: table-cell;\n  float: none;\n  width: 1%;\n}\n.btn-group-justified > .btn-group .btn {\n  width: 100%;\n}\n[data-toggle=\"buttons\"] > .btn > input[type=\"radio\"],\n[data-toggle=\"buttons\"] > .btn > input[type=\"checkbox\"] {\n  display: none;\n}\n.input-group {\n  position: relative;\n  display: table;\n  border-collapse: separate;\n}\n.input-group[class*=\"col-\"] {\n  float: none;\n  padding-right: 0;\n  padding-left: 0;\n}\n.input-group .form-control {\n  position: relative;\n  z-index: 2;\n  float: left;\n  width: 100%;\n  margin-bottom: 0;\n}\n.input-group-lg > .form-control,\n.input-group-lg > .input-group-addon,\n.input-group-lg > .input-group-btn > .btn {\n  height: 46px;\n  padding: 10px 16px;\n  font-size: 18px;\n  line-height: 1.33;\n  border-radius: 6px;\n}\nselect.input-group-lg > .form-control,\nselect.input-group-lg > .input-group-addon,\nselect.input-group-lg > .input-group-btn > .btn {\n  height: 46px;\n  line-height: 46px;\n}\ntextarea.input-group-lg > .form-control,\ntextarea.input-group-lg > .input-group-addon,\ntextarea.input-group-lg > .input-group-btn > .btn,\nselect[multiple].input-group-lg > .form-control,\nselect[multiple].input-group-lg > .input-group-addon,\nselect[multiple].input-group-lg > .input-group-btn > .btn {\n  height: auto;\n}\n.input-group-sm > .form-control,\n.input-group-sm > .input-group-addon,\n.input-group-sm > .input-group-btn > .btn {\n  height: 30px;\n  padding: 5px 10px;\n  font-size: 12px;\n  line-height: 1.5;\n  border-radius: 3px;\n}\nselect.input-group-sm > .form-control,\nselect.input-group-sm > .input-group-addon,\nselect.input-group-sm > .input-group-btn > .btn {\n  height: 30px;\n  line-height: 30px;\n}\ntextarea.input-group-sm > .form-control,\ntextarea.input-group-sm > .input-group-addon,\ntextarea.input-group-sm > .input-group-btn > .btn,\nselect[multiple].input-group-sm > .form-control,\nselect[multiple].input-group-sm > .input-group-addon,\nselect[multiple].input-group-sm > .input-group-btn > .btn {\n  height: auto;\n}\n.input-group-addon,\n.input-group-btn,\n.input-group .form-control {\n  display: table-cell;\n}\n.input-group-addon:not(:first-child):not(:last-child),\n.input-group-btn:not(:first-child):not(:last-child),\n.input-group .form-control:not(:first-child):not(:last-child) {\n  border-radius: 0;\n}\n.input-group-addon,\n.input-group-btn {\n  width: 1%;\n  white-space: nowrap;\n  vertical-align: middle;\n}\n.input-group-addon {\n  padding: 6px 12px;\n  font-size: 14px;\n  font-weight: normal;\n  line-height: 1;\n  color: #555;\n  text-align: center;\n  background-color: #eee;\n  border: 1px solid #ccc;\n  border-radius: 4px;\n}\n.input-group-addon.input-sm {\n  padding: 5px 10px;\n  font-size: 12px;\n  border-radius: 3px;\n}\n.input-group-addon.input-lg {\n  padding: 10px 16px;\n  font-size: 18px;\n  border-radius: 6px;\n}\n.input-group-addon input[type=\"radio\"],\n.input-group-addon input[type=\"checkbox\"] {\n  margin-top: 0;\n}\n.input-group .form-control:first-child,\n.input-group-addon:first-child,\n.input-group-btn:first-child > .btn,\n.input-group-btn:first-child > .btn-group > .btn,\n.input-group-btn:first-child > .dropdown-toggle,\n.input-group-btn:last-child > .btn:not(:last-child):not(.dropdown-toggle),\n.input-group-btn:last-child > .btn-group:not(:last-child) > .btn {\n  border-top-right-radius: 0;\n  border-bottom-right-radius: 0;\n}\n.input-group-addon:first-child {\n  border-right: 0;\n}\n.input-group .form-control:last-child,\n.input-group-addon:last-child,\n.input-group-btn:last-child > .btn,\n.input-group-btn:last-child > .btn-group > .btn,\n.input-group-btn:last-child > .dropdown-toggle,\n.input-group-btn:first-child > .btn:not(:first-child),\n.input-group-btn:first-child > .btn-group:not(:first-child) > .btn {\n  border-top-left-radius: 0;\n  border-bottom-left-radius: 0;\n}\n.input-group-addon:last-child {\n  border-left: 0;\n}\n.input-group-btn {\n  position: relative;\n  font-size: 0;\n  white-space: nowrap;\n}\n.input-group-btn > .btn {\n  position: relative;\n}\n.input-group-btn > .btn + .btn {\n  margin-left: -1px;\n}\n.input-group-btn > .btn:hover,\n.input-group-btn > .btn:focus,\n.input-group-btn > .btn:active {\n  z-index: 2;\n}\n.input-group-btn:first-child > .btn,\n.input-group-btn:first-child > .btn-group {\n  margin-right: -1px;\n}\n.input-group-btn:last-child > .btn,\n.input-group-btn:last-child > .btn-group {\n  margin-left: -1px;\n}\n.nav {\n  padding-left: 0;\n  margin-bottom: 0;\n  list-style: none;\n}\n.nav > li {\n  position: relative;\n  display: block;\n}\n.nav > li > a {\n  position: relative;\n  display: block;\n  padding: 10px 15px;\n}\n.nav > li > a:hover,\n.nav > li > a:focus {\n  text-decoration: none;\n  background-color: #eee;\n}\n.nav > li.disabled > a {\n  color: #999;\n}\n.nav > li.disabled > a:hover,\n.nav > li.disabled > a:focus {\n  color: #999;\n  text-decoration: none;\n  cursor: not-allowed;\n  background-color: transparent;\n}\n.nav .open > a,\n.nav .open > a:hover,\n.nav .open > a:focus {\n  background-color: #eee;\n  border-color: #428bca;\n}\n.nav .nav-divider {\n  height: 1px;\n  margin: 9px 0;\n  overflow: hidden;\n  background-color: #e5e5e5;\n}\n.nav > li > a > img {\n  max-width: none;\n}\n.nav-tabs {\n  border-bottom: 1px solid #ddd;\n}\n.nav-tabs > li {\n  float: left;\n  margin-bottom: -1px;\n}\n.nav-tabs > li > a {\n  margin-right: 2px;\n  line-height: 1.42857143;\n  border: 1px solid transparent;\n  border-radius: 4px 4px 0 0;\n}\n.nav-tabs > li > a:hover {\n  border-color: #eee #eee #ddd;\n}\n.nav-tabs > li.active > a,\n.nav-tabs > li.active > a:hover,\n.nav-tabs > li.active > a:focus {\n  color: #555;\n  cursor: default;\n  background-color: #fff;\n  border: 1px solid #ddd;\n  border-bottom-color: transparent;\n}\n.nav-tabs.nav-justified {\n  width: 100%;\n  border-bottom: 0;\n}\n.nav-tabs.nav-justified > li {\n  float: none;\n}\n.nav-tabs.nav-justified > li > a {\n  margin-bottom: 5px;\n  text-align: center;\n}\n.nav-tabs.nav-justified > .dropdown .dropdown-menu {\n  top: auto;\n  left: auto;\n}\n@media (min-width: 768px) {\n  .nav-tabs.nav-justified > li {\n    display: table-cell;\n    width: 1%;\n  }\n  .nav-tabs.nav-justified > li > a {\n    margin-bottom: 0;\n  }\n}\n.nav-tabs.nav-justified > li > a {\n  margin-right: 0;\n  border-radius: 4px;\n}\n.nav-tabs.nav-justified > .active > a,\n.nav-tabs.nav-justified > .active > a:hover,\n.nav-tabs.nav-justified > .active > a:focus {\n  border: 1px solid #ddd;\n}\n@media (min-width: 768px) {\n  .nav-tabs.nav-justified > li > a {\n    border-bottom: 1px solid #ddd;\n    border-radius: 4px 4px 0 0;\n  }\n  .nav-tabs.nav-justified > .active > a,\n  .nav-tabs.nav-justified > .active > a:hover,\n  .nav-tabs.nav-justified > .active > a:focus {\n    border-bottom-color: #fff;\n  }\n}\n.nav-pills > li {\n  float: left;\n}\n.nav-pills > li > a {\n  border-radius: 4px;\n}\n.nav-pills > li + li {\n  margin-left: 2px;\n}\n.nav-pills > li.active > a,\n.nav-pills > li.active > a:hover,\n.nav-pills > li.active > a:focus {\n  color: #fff;\n  background-color: #428bca;\n}\n.nav-stacked > li {\n  float: none;\n}\n.nav-stacked > li + li {\n  margin-top: 2px;\n  margin-left: 0;\n}\n.nav-justified {\n  width: 100%;\n}\n.nav-justified > li {\n  float: none;\n}\n.nav-justified > li > a {\n  margin-bottom: 5px;\n  text-align: center;\n}\n.nav-justified > .dropdown .dropdown-menu {\n  top: auto;\n  left: auto;\n}\n@media (min-width: 768px) {\n  .nav-justified > li {\n    display: table-cell;\n    width: 1%;\n  }\n  .nav-justified > li > a {\n    margin-bottom: 0;\n  }\n}\n.nav-tabs-justified {\n  border-bottom: 0;\n}\n.nav-tabs-justified > li > a {\n  margin-right: 0;\n  border-radius: 4px;\n}\n.nav-tabs-justified > .active > a,\n.nav-tabs-justified > .active > a:hover,\n.nav-tabs-justified > .active > a:focus {\n  border: 1px solid #ddd;\n}\n@media (min-width: 768px) {\n  .nav-tabs-justified > li > a {\n    border-bottom: 1px solid #ddd;\n    border-radius: 4px 4px 0 0;\n  }\n  .nav-tabs-justified > .active > a,\n  .nav-tabs-justified > .active > a:hover,\n  .nav-tabs-justified > .active > a:focus {\n    border-bottom-color: #fff;\n  }\n}\n.tab-content > .tab-pane {\n  display: none;\n}\n.tab-content > .active {\n  display: block;\n}\n.nav-tabs .dropdown-menu {\n  margin-top: -1px;\n  border-top-left-radius: 0;\n  border-top-right-radius: 0;\n}\n.navbar {\n  position: relative;\n  min-height: 50px;\n  margin-bottom: 20px;\n  border: 1px solid transparent;\n}\n@media (min-width: 768px) {\n  .navbar {\n    border-radius: 4px;\n  }\n}\n@media (min-width: 768px) {\n  .navbar-header {\n    float: left;\n  }\n}\n.navbar-collapse {\n  max-height: 340px;\n  padding-right: 15px;\n  padding-left: 15px;\n  overflow-x: visible;\n  -webkit-overflow-scrolling: touch;\n  border-top: 1px solid transparent;\n  box-shadow: inset 0 1px 0 rgba(255, 255, 255, .1);\n}\n.navbar-collapse.in {\n  overflow-y: auto;\n}\n@media (min-width: 768px) {\n  .navbar-collapse {\n    width: auto;\n    border-top: 0;\n    box-shadow: none;\n  }\n  .navbar-collapse.collapse {\n    display: block !important;\n    height: auto !important;\n    padding-bottom: 0;\n    overflow: visible !important;\n  }\n  .navbar-collapse.in {\n    overflow-y: visible;\n  }\n  .navbar-fixed-top .navbar-collapse,\n  .navbar-static-top .navbar-collapse,\n  .navbar-fixed-bottom .navbar-collapse {\n    padding-right: 0;\n    padding-left: 0;\n  }\n}\n.container > .navbar-header,\n.container-fluid > .navbar-header,\n.container > .navbar-collapse,\n.container-fluid > .navbar-collapse {\n  margin-right: -15px;\n  margin-left: -15px;\n}\n@media (min-width: 768px) {\n  .container > .navbar-header,\n  .container-fluid > .navbar-header,\n  .container > .navbar-collapse,\n  .container-fluid > .navbar-collapse {\n    margin-right: 0;\n    margin-left: 0;\n  }\n}\n.navbar-static-top {\n  z-index: 1000;\n  border-width: 0 0 1px;\n}\n@media (min-width: 768px) {\n  .navbar-static-top {\n    border-radius: 0;\n  }\n}\n.navbar-fixed-top,\n.navbar-fixed-bottom {\n  position: fixed;\n  right: 0;\n  left: 0;\n  z-index: 1030;\n}\n@media (min-width: 768px) {\n  .navbar-fixed-top,\n  .navbar-fixed-bottom {\n    border-radius: 0;\n  }\n}\n.navbar-fixed-top {\n  top: 0;\n  border-width: 0 0 1px;\n}\n.navbar-fixed-bottom {\n  bottom: 0;\n  margin-bottom: 0;\n  border-width: 1px 0 0;\n}\n.navbar-brand {\n  float: left;\n  height: 50px;\n  padding: 15px 15px;\n  font-size: 18px;\n  line-height: 20px;\n}\n.navbar-brand:hover,\n.navbar-brand:focus {\n  text-decoration: none;\n}\n@media (min-width: 768px) {\n  .navbar > .container .navbar-brand,\n  .navbar > .container-fluid .navbar-brand {\n    margin-left: -15px;\n  }\n}\n.navbar-toggle {\n  position: relative;\n  float: right;\n  padding: 9px 10px;\n  margin-top: 8px;\n  margin-right: 15px;\n  margin-bottom: 8px;\n  background-color: transparent;\n  background-image: none;\n  border: 1px solid transparent;\n  border-radius: 4px;\n}\n.navbar-toggle:focus {\n  outline: none;\n}\n.navbar-toggle .icon-bar {\n  display: block;\n  width: 22px;\n  height: 2px;\n  border-radius: 1px;\n}\n.navbar-toggle .icon-bar + .icon-bar {\n  margin-top: 4px;\n}\n@media (min-width: 768px) {\n  .navbar-toggle {\n    display: none;\n  }\n}\n.navbar-nav {\n  margin: 7.5px -15px;\n}\n.navbar-nav > li > a {\n  padding-top: 10px;\n  padding-bottom: 10px;\n  line-height: 20px;\n}\n@media (max-width: 767px) {\n  .navbar-nav .open .dropdown-menu {\n    position: static;\n    float: none;\n    width: auto;\n    margin-top: 0;\n    background-color: transparent;\n    border: 0;\n    box-shadow: none;\n  }\n  .navbar-nav .open .dropdown-menu > li > a,\n  .navbar-nav .open .dropdown-menu .dropdown-header {\n    padding: 5px 15px 5px 25px;\n  }\n  .navbar-nav .open .dropdown-menu > li > a {\n    line-height: 20px;\n  }\n  .navbar-nav .open .dropdown-menu > li > a:hover,\n  .navbar-nav .open .dropdown-menu > li > a:focus {\n    background-image: none;\n  }\n}\n@media (min-width: 768px) {\n  .navbar-nav {\n    float: left;\n    margin: 0;\n  }\n  .navbar-nav > li {\n    float: left;\n  }\n  .navbar-nav > li > a {\n    padding-top: 15px;\n    padding-bottom: 15px;\n  }\n  .navbar-nav.navbar-right:last-child {\n    margin-right: -15px;\n  }\n}\n@media (min-width: 768px) {\n  .navbar-left {\n    float: left !important;\n  }\n  .navbar-right {\n    float: right !important;\n  }\n}\n.navbar-form {\n  padding: 10px 15px;\n  margin-top: 8px;\n  margin-right: -15px;\n  margin-bottom: 8px;\n  margin-left: -15px;\n  border-top: 1px solid transparent;\n  border-bottom: 1px solid transparent;\n  -webkit-box-shadow: inset 0 1px 0 rgba(255, 255, 255, .1), 0 1px 0 rgba(255, 255, 255, .1);\n          box-shadow: inset 0 1px 0 rgba(255, 255, 255, .1), 0 1px 0 rgba(255, 255, 255, .1);\n}\n@media (min-width: 768px) {\n  .navbar-form .form-group {\n    display: inline-block;\n    margin-bottom: 0;\n    vertical-align: middle;\n  }\n  .navbar-form .form-control {\n    display: inline-block;\n    width: auto;\n    vertical-align: middle;\n  }\n  .navbar-form .input-group > .form-control {\n    width: 100%;\n  }\n  .navbar-form .control-label {\n    margin-bottom: 0;\n    vertical-align: middle;\n  }\n  .navbar-form .radio,\n  .navbar-form .checkbox {\n    display: inline-block;\n    padding-left: 0;\n    margin-top: 0;\n    margin-bottom: 0;\n    vertical-align: middle;\n  }\n  .navbar-form .radio input[type=\"radio\"],\n  .navbar-form .checkbox input[type=\"checkbox\"] {\n    float: none;\n    margin-left: 0;\n  }\n  .navbar-form .has-feedback .form-control-feedback {\n    top: 0;\n  }\n}\n@media (max-width: 767px) {\n  .navbar-form .form-group {\n    margin-bottom: 5px;\n  }\n}\n@media (min-width: 768px) {\n  .navbar-form {\n    width: auto;\n    padding-top: 0;\n    padding-bottom: 0;\n    margin-right: 0;\n    margin-left: 0;\n    border: 0;\n    -webkit-box-shadow: none;\n            box-shadow: none;\n  }\n  .navbar-form.navbar-right:last-child {\n    margin-right: -15px;\n  }\n}\n.navbar-nav > li > .dropdown-menu {\n  margin-top: 0;\n  border-top-left-radius: 0;\n  border-top-right-radius: 0;\n}\n.navbar-fixed-bottom .navbar-nav > li > .dropdown-menu {\n  border-bottom-right-radius: 0;\n  border-bottom-left-radius: 0;\n}\n.navbar-btn {\n  margin-top: 8px;\n  margin-bottom: 8px;\n}\n.navbar-btn.btn-sm {\n  margin-top: 10px;\n  margin-bottom: 10px;\n}\n.navbar-btn.btn-xs {\n  margin-top: 14px;\n  margin-bottom: 14px;\n}\n.navbar-text {\n  margin-top: 15px;\n  margin-bottom: 15px;\n}\n@media (min-width: 768px) {\n  .navbar-text {\n    float: left;\n    margin-right: 15px;\n    margin-left: 15px;\n  }\n  .navbar-text.navbar-right:last-child {\n    margin-right: 0;\n  }\n}\n.navbar-default {\n  background-color: #f8f8f8;\n  border-color: #e7e7e7;\n}\n.navbar-default .navbar-brand {\n  color: #777;\n}\n.navbar-default .navbar-brand:hover,\n.navbar-default .navbar-brand:focus {\n  color: #5e5e5e;\n  background-color: transparent;\n}\n.navbar-default .navbar-text {\n  color: #777;\n}\n.navbar-default .navbar-nav > li > a {\n  color: #777;\n}\n.navbar-default .navbar-nav > li > a:hover,\n.navbar-default .navbar-nav > li > a:focus {\n  color: #333;\n  background-color: transparent;\n}\n.navbar-default .navbar-nav > .active > a,\n.navbar-default .navbar-nav > .active > a:hover,\n.navbar-default .navbar-nav > .active > a:focus {\n  color: #555;\n  background-color: #e7e7e7;\n}\n.navbar-default .navbar-nav > .disabled > a,\n.navbar-default .navbar-nav > .disabled > a:hover,\n.navbar-default .navbar-nav > .disabled > a:focus {\n  color: #ccc;\n  background-color: transparent;\n}\n.navbar-default .navbar-toggle {\n  border-color: #ddd;\n}\n.navbar-default .navbar-toggle:hover,\n.navbar-default .navbar-toggle:focus {\n  background-color: #ddd;\n}\n.navbar-default .navbar-toggle .icon-bar {\n  background-color: #888;\n}\n.navbar-default .navbar-collapse,\n.navbar-default .navbar-form {\n  border-color: #e7e7e7;\n}\n.navbar-default .navbar-nav > .open > a,\n.navbar-default .navbar-nav > .open > a:hover,\n.navbar-default .navbar-nav > .open > a:focus {\n  color: #555;\n  background-color: #e7e7e7;\n}\n@media (max-width: 767px) {\n  .navbar-default .navbar-nav .open .dropdown-menu > li > a {\n    color: #777;\n  }\n  .navbar-default .navbar-nav .open .dropdown-menu > li > a:hover,\n  .navbar-default .navbar-nav .open .dropdown-menu > li > a:focus {\n    color: #333;\n    background-color: transparent;\n  }\n  .navbar-default .navbar-nav .open .dropdown-menu > .active > a,\n  .navbar-default .navbar-nav .open .dropdown-menu > .active > a:hover,\n  .navbar-default .navbar-nav .open .dropdown-menu > .active > a:focus {\n    color: #555;\n    background-color: #e7e7e7;\n  }\n  .navbar-default .navbar-nav .open .dropdown-menu > .disabled > a,\n  .navbar-default .navbar-nav .open .dropdown-menu > .disabled > a:hover,\n  .navbar-default .navbar-nav .open .dropdown-menu > .disabled > a:focus {\n    color: #ccc;\n    background-color: transparent;\n  }\n}\n.navbar-default .navbar-link {\n  color: #777;\n}\n.navbar-default .navbar-link:hover {\n  color: #333;\n}\n.navbar-inverse {\n  background-color: #222;\n  border-color: #080808;\n}\n.navbar-inverse .navbar-brand {\n  color: #999;\n}\n.navbar-inverse .navbar-brand:hover,\n.navbar-inverse .navbar-brand:focus {\n  color: #fff;\n  background-color: transparent;\n}\n.navbar-inverse .navbar-text {\n  color: #999;\n}\n.navbar-inverse .navbar-nav > li > a {\n  color: #999;\n}\n.navbar-inverse .navbar-nav > li > a:hover,\n.navbar-inverse .navbar-nav > li > a:focus {\n  color: #fff;\n  background-color: transparent;\n}\n.navbar-inverse .navbar-nav > .active > a,\n.navbar-inverse .navbar-nav > .active > a:hover,\n.navbar-inverse .navbar-nav > .active > a:focus {\n  color: #fff;\n  background-color: #080808;\n}\n.navbar-inverse .navbar-nav > .disabled > a,\n.navbar-inverse .navbar-nav > .disabled > a:hover,\n.navbar-inverse .navbar-nav > .disabled > a:focus {\n  color: #444;\n  background-color: transparent;\n}\n.navbar-inverse .navbar-toggle {\n  border-color: #333;\n}\n.navbar-inverse .navbar-toggle:hover,\n.navbar-inverse .navbar-toggle:focus {\n  background-color: #333;\n}\n.navbar-inverse .navbar-toggle .icon-bar {\n  background-color: #fff;\n}\n.navbar-inverse .navbar-collapse,\n.navbar-inverse .navbar-form {\n  border-color: #101010;\n}\n.navbar-inverse .navbar-nav > .open > a,\n.navbar-inverse .navbar-nav > .open > a:hover,\n.navbar-inverse .navbar-nav > .open > a:focus {\n  color: #fff;\n  background-color: #080808;\n}\n@media (max-width: 767px) {\n  .navbar-inverse .navbar-nav .open .dropdown-menu > .dropdown-header {\n    border-color: #080808;\n  }\n  .navbar-inverse .navbar-nav .open .dropdown-menu .divider {\n    background-color: #080808;\n  }\n  .navbar-inverse .navbar-nav .open .dropdown-menu > li > a {\n    color: #999;\n  }\n  .navbar-inverse .navbar-nav .open .dropdown-menu > li > a:hover,\n  .navbar-inverse .navbar-nav .open .dropdown-menu > li > a:focus {\n    color: #fff;\n    background-color: transparent;\n  }\n  .navbar-inverse .navbar-nav .open .dropdown-menu > .active > a,\n  .navbar-inverse .navbar-nav .open .dropdown-menu > .active > a:hover,\n  .navbar-inverse .navbar-nav .open .dropdown-menu > .active > a:focus {\n    color: #fff;\n    background-color: #080808;\n  }\n  .navbar-inverse .navbar-nav .open .dropdown-menu > .disabled > a,\n  .navbar-inverse .navbar-nav .open .dropdown-menu > .disabled > a:hover,\n  .navbar-inverse .navbar-nav .open .dropdown-menu > .disabled > a:focus {\n    color: #444;\n    background-color: transparent;\n  }\n}\n.navbar-inverse .navbar-link {\n  color: #999;\n}\n.navbar-inverse .navbar-link:hover {\n  color: #fff;\n}\n.breadcrumb {\n  padding: 8px 15px;\n  margin-bottom: 20px;\n  list-style: none;\n  background-color: #f5f5f5;\n  border-radius: 4px;\n}\n.breadcrumb > li {\n  display: inline-block;\n}\n.breadcrumb > li + li:before {\n  padding: 0 5px;\n  color: #ccc;\n  content: \"/\\00a0\";\n}\n.breadcrumb > .active {\n  color: #999;\n}\n.pagination {\n  display: inline-block;\n  padding-left: 0;\n  margin: 20px 0;\n  border-radius: 4px;\n}\n.pagination > li {\n  display: inline;\n}\n.pagination > li > a,\n.pagination > li > span {\n  position: relative;\n  float: left;\n  padding: 6px 12px;\n  margin-left: -1px;\n  line-height: 1.42857143;\n  color: #428bca;\n  text-decoration: none;\n  background-color: #fff;\n  border: 1px solid #ddd;\n}\n.pagination > li:first-child > a,\n.pagination > li:first-child > span {\n  margin-left: 0;\n  border-top-left-radius: 4px;\n  border-bottom-left-radius: 4px;\n}\n.pagination > li:last-child > a,\n.pagination > li:last-child > span {\n  border-top-right-radius: 4px;\n  border-bottom-right-radius: 4px;\n}\n.pagination > li > a:hover,\n.pagination > li > span:hover,\n.pagination > li > a:focus,\n.pagination > li > span:focus {\n  color: #2a6496;\n  background-color: #eee;\n  border-color: #ddd;\n}\n.pagination > .active > a,\n.pagination > .active > span,\n.pagination > .active > a:hover,\n.pagination > .active > span:hover,\n.pagination > .active > a:focus,\n.pagination > .active > span:focus {\n  z-index: 2;\n  color: #fff;\n  cursor: default;\n  background-color: #428bca;\n  border-color: #428bca;\n}\n.pagination > .disabled > span,\n.pagination > .disabled > span:hover,\n.pagination > .disabled > span:focus,\n.pagination > .disabled > a,\n.pagination > .disabled > a:hover,\n.pagination > .disabled > a:focus {\n  color: #999;\n  cursor: not-allowed;\n  background-color: #fff;\n  border-color: #ddd;\n}\n.pagination-lg > li > a,\n.pagination-lg > li > span {\n  padding: 10px 16px;\n  font-size: 18px;\n}\n.pagination-lg > li:first-child > a,\n.pagination-lg > li:first-child > span {\n  border-top-left-radius: 6px;\n  border-bottom-left-radius: 6px;\n}\n.pagination-lg > li:last-child > a,\n.pagination-lg > li:last-child > span {\n  border-top-right-radius: 6px;\n  border-bottom-right-radius: 6px;\n}\n.pagination-sm > li > a,\n.pagination-sm > li > span {\n  padding: 5px 10px;\n  font-size: 12px;\n}\n.pagination-sm > li:first-child > a,\n.pagination-sm > li:first-child > span {\n  border-top-left-radius: 3px;\n  border-bottom-left-radius: 3px;\n}\n.pagination-sm > li:last-child > a,\n.pagination-sm > li:last-child > span {\n  border-top-right-radius: 3px;\n  border-bottom-right-radius: 3px;\n}\n.pager {\n  padding-left: 0;\n  margin: 20px 0;\n  text-align: center;\n  list-style: none;\n}\n.pager li {\n  display: inline;\n}\n.pager li > a,\n.pager li > span {\n  display: inline-block;\n  padding: 5px 14px;\n  background-color: #fff;\n  border: 1px solid #ddd;\n  border-radius: 15px;\n}\n.pager li > a:hover,\n.pager li > a:focus {\n  text-decoration: none;\n  background-color: #eee;\n}\n.pager .next > a,\n.pager .next > span {\n  float: right;\n}\n.pager .previous > a,\n.pager .previous > span {\n  float: left;\n}\n.pager .disabled > a,\n.pager .disabled > a:hover,\n.pager .disabled > a:focus,\n.pager .disabled > span {\n  color: #999;\n  cursor: not-allowed;\n  background-color: #fff;\n}\n.label {\n  display: inline;\n  padding: .2em .6em .3em;\n  font-size: 75%;\n  font-weight: bold;\n  line-height: 1;\n  color: #fff;\n  text-align: center;\n  white-space: nowrap;\n  vertical-align: baseline;\n  border-radius: .25em;\n}\n.label[href]:hover,\n.label[href]:focus {\n  color: #fff;\n  text-decoration: none;\n  cursor: pointer;\n}\n.label:empty {\n  display: none;\n}\n.btn .label {\n  position: relative;\n  top: -1px;\n}\n.label-default {\n  background-color: #999;\n}\n.label-default[href]:hover,\n.label-default[href]:focus {\n  background-color: #808080;\n}\n.label-primary {\n  background-color: #428bca;\n}\n.label-primary[href]:hover,\n.label-primary[href]:focus {\n  background-color: #3071a9;\n}\n.label-success {\n  background-color: #5cb85c;\n}\n.label-success[href]:hover,\n.label-success[href]:focus {\n  background-color: #449d44;\n}\n.label-info {\n  background-color: #5bc0de;\n}\n.label-info[href]:hover,\n.label-info[href]:focus {\n  background-color: #31b0d5;\n}\n.label-warning {\n  background-color: #f0ad4e;\n}\n.label-warning[href]:hover,\n.label-warning[href]:focus {\n  background-color: #ec971f;\n}\n.label-danger {\n  background-color: #d9534f;\n}\n.label-danger[href]:hover,\n.label-danger[href]:focus {\n  background-color: #c9302c;\n}\n.badge {\n  display: inline-block;\n  min-width: 10px;\n  padding: 3px 7px;\n  font-size: 12px;\n  font-weight: bold;\n  line-height: 1;\n  color: #fff;\n  text-align: center;\n  white-space: nowrap;\n  vertical-align: baseline;\n  background-color: #999;\n  border-radius: 10px;\n}\n.badge:empty {\n  display: none;\n}\n.btn .badge {\n  position: relative;\n  top: -1px;\n}\n.btn-xs .badge {\n  top: 0;\n  padding: 1px 5px;\n}\na.badge:hover,\na.badge:focus {\n  color: #fff;\n  text-decoration: none;\n  cursor: pointer;\n}\na.list-group-item.active > .badge,\n.nav-pills > .active > a > .badge {\n  color: #428bca;\n  background-color: #fff;\n}\n.nav-pills > li > a > .badge {\n  margin-left: 3px;\n}\n.jumbotron {\n  padding: 30px;\n  margin-bottom: 30px;\n  color: inherit;\n  background-color: #eee;\n}\n.jumbotron h1,\n.jumbotron .h1 {\n  color: inherit;\n}\n.jumbotron p {\n  margin-bottom: 15px;\n  font-size: 21px;\n  font-weight: 200;\n}\n.container .jumbotron {\n  border-radius: 6px;\n}\n.jumbotron .container {\n  max-width: 100%;\n}\n@media screen and (min-width: 768px) {\n  .jumbotron {\n    padding-top: 48px;\n    padding-bottom: 48px;\n  }\n  .container .jumbotron {\n    padding-right: 60px;\n    padding-left: 60px;\n  }\n  .jumbotron h1,\n  .jumbotron .h1 {\n    font-size: 63px;\n  }\n}\n.thumbnail {\n  display: block;\n  padding: 4px;\n  margin-bottom: 20px;\n  line-height: 1.42857143;\n  background-color: #fff;\n  border: 1px solid #ddd;\n  border-radius: 4px;\n  -webkit-transition: all .2s ease-in-out;\n          transition: all .2s ease-in-out;\n}\n.thumbnail > img,\n.thumbnail a > img {\n  margin-right: auto;\n  margin-left: auto;\n}\na.thumbnail:hover,\na.thumbnail:focus,\na.thumbnail.active {\n  border-color: #428bca;\n}\n.thumbnail .caption {\n  padding: 9px;\n  color: #333;\n}\n.alert {\n  padding: 15px;\n  margin-bottom: 20px;\n  border: 1px solid transparent;\n  border-radius: 4px;\n}\n.alert h4 {\n  margin-top: 0;\n  color: inherit;\n}\n.alert .alert-link {\n  font-weight: bold;\n}\n.alert > p,\n.alert > ul {\n  margin-bottom: 0;\n}\n.alert > p + p {\n  margin-top: 5px;\n}\n.alert-dismissable {\n  padding-right: 35px;\n}\n.alert-dismissable .close {\n  position: relative;\n  top: -2px;\n  right: -21px;\n  color: inherit;\n}\n.alert-success {\n  color: #3c763d;\n  background-color: #dff0d8;\n  border-color: #d6e9c6;\n}\n.alert-success hr {\n  border-top-color: #c9e2b3;\n}\n.alert-success .alert-link {\n  color: #2b542c;\n}\n.alert-info {\n  color: #31708f;\n  background-color: #d9edf7;\n  border-color: #bce8f1;\n}\n.alert-info hr {\n  border-top-color: #a6e1ec;\n}\n.alert-info .alert-link {\n  color: #245269;\n}\n.alert-warning {\n  color: #8a6d3b;\n  background-color: #fcf8e3;\n  border-color: #faebcc;\n}\n.alert-warning hr {\n  border-top-color: #f7e1b5;\n}\n.alert-warning .alert-link {\n  color: #66512c;\n}\n.alert-danger {\n  color: #a94442;\n  background-color: #f2dede;\n  border-color: #ebccd1;\n}\n.alert-danger hr {\n  border-top-color: #e4b9c0;\n}\n.alert-danger .alert-link {\n  color: #843534;\n}\n@-webkit-keyframes progress-bar-stripes {\n  from {\n    background-position: 40px 0;\n  }\n  to {\n    background-position: 0 0;\n  }\n}\n@keyframes progress-bar-stripes {\n  from {\n    background-position: 40px 0;\n  }\n  to {\n    background-position: 0 0;\n  }\n}\n.progress {\n  height: 20px;\n  margin-bottom: 20px;\n  overflow: hidden;\n  background-color: #f5f5f5;\n  border-radius: 4px;\n  -webkit-box-shadow: inset 0 1px 2px rgba(0, 0, 0, .1);\n          box-shadow: inset 0 1px 2px rgba(0, 0, 0, .1);\n}\n.progress-bar {\n  float: left;\n  width: 0;\n  height: 100%;\n  font-size: 12px;\n  line-height: 20px;\n  color: #fff;\n  text-align: center;\n  background-color: #428bca;\n  -webkit-box-shadow: inset 0 -1px 0 rgba(0, 0, 0, .15);\n          box-shadow: inset 0 -1px 0 rgba(0, 0, 0, .15);\n  -webkit-transition: width .6s ease;\n          transition: width .6s ease;\n}\n.progress-striped .progress-bar {\n  background-image: -webkit-linear-gradient(45deg, rgba(255, 255, 255, .15) 25%, transparent 25%, transparent 50%, rgba(255, 255, 255, .15) 50%, rgba(255, 255, 255, .15) 75%, transparent 75%, transparent);\n  background-image:         linear-gradient(45deg, rgba(255, 255, 255, .15) 25%, transparent 25%, transparent 50%, rgba(255, 255, 255, .15) 50%, rgba(255, 255, 255, .15) 75%, transparent 75%, transparent);\n  background-size: 40px 40px;\n}\n.progress.active .progress-bar {\n  -webkit-animation: progress-bar-stripes 2s linear infinite;\n          animation: progress-bar-stripes 2s linear infinite;\n}\n.progress-bar-success {\n  background-color: #5cb85c;\n}\n.progress-striped .progress-bar-success {\n  background-image: -webkit-linear-gradient(45deg, rgba(255, 255, 255, .15) 25%, transparent 25%, transparent 50%, rgba(255, 255, 255, .15) 50%, rgba(255, 255, 255, .15) 75%, transparent 75%, transparent);\n  background-image:         linear-gradient(45deg, rgba(255, 255, 255, .15) 25%, transparent 25%, transparent 50%, rgba(255, 255, 255, .15) 50%, rgba(255, 255, 255, .15) 75%, transparent 75%, transparent);\n}\n.progress-bar-info {\n  background-color: #5bc0de;\n}\n.progress-striped .progress-bar-info {\n  background-image: -webkit-linear-gradient(45deg, rgba(255, 255, 255, .15) 25%, transparent 25%, transparent 50%, rgba(255, 255, 255, .15) 50%, rgba(255, 255, 255, .15) 75%, transparent 75%, transparent);\n  background-image:         linear-gradient(45deg, rgba(255, 255, 255, .15) 25%, transparent 25%, transparent 50%, rgba(255, 255, 255, .15) 50%, rgba(255, 255, 255, .15) 75%, transparent 75%, transparent);\n}\n.progress-bar-warning {\n  background-color: #f0ad4e;\n}\n.progress-striped .progress-bar-warning {\n  background-image: -webkit-linear-gradient(45deg, rgba(255, 255, 255, .15) 25%, transparent 25%, transparent 50%, rgba(255, 255, 255, .15) 50%, rgba(255, 255, 255, .15) 75%, transparent 75%, transparent);\n  background-image:         linear-gradient(45deg, rgba(255, 255, 255, .15) 25%, transparent 25%, transparent 50%, rgba(255, 255, 255, .15) 50%, rgba(255, 255, 255, .15) 75%, transparent 75%, transparent);\n}\n.progress-bar-danger {\n  background-color: #d9534f;\n}\n.progress-striped .progress-bar-danger {\n  background-image: -webkit-linear-gradient(45deg, rgba(255, 255, 255, .15) 25%, transparent 25%, transparent 50%, rgba(255, 255, 255, .15) 50%, rgba(255, 255, 255, .15) 75%, transparent 75%, transparent);\n  background-image:         linear-gradient(45deg, rgba(255, 255, 255, .15) 25%, transparent 25%, transparent 50%, rgba(255, 255, 255, .15) 50%, rgba(255, 255, 255, .15) 75%, transparent 75%, transparent);\n}\n.media,\n.media-body {\n  overflow: hidden;\n  zoom: 1;\n}\n.media,\n.media .media {\n  margin-top: 15px;\n}\n.media:first-child {\n  margin-top: 0;\n}\n.media-object {\n  display: block;\n}\n.media-heading {\n  margin: 0 0 5px;\n}\n.media > .pull-left {\n  margin-right: 10px;\n}\n.media > .pull-right {\n  margin-left: 10px;\n}\n.media-list {\n  padding-left: 0;\n  list-style: none;\n}\n.list-group {\n  padding-left: 0;\n  margin-bottom: 20px;\n}\n.list-group-item {\n  position: relative;\n  display: block;\n  padding: 10px 15px;\n  margin-bottom: -1px;\n  background-color: #fff;\n  border: 1px solid #ddd;\n}\n.list-group-item:first-child {\n  border-top-left-radius: 4px;\n  border-top-right-radius: 4px;\n}\n.list-group-item:last-child {\n  margin-bottom: 0;\n  border-bottom-right-radius: 4px;\n  border-bottom-left-radius: 4px;\n}\n.list-group-item > .badge {\n  float: right;\n}\n.list-group-item > .badge + .badge {\n  margin-right: 5px;\n}\na.list-group-item {\n  color: #555;\n}\na.list-group-item .list-group-item-heading {\n  color: #333;\n}\na.list-group-item:hover,\na.list-group-item:focus {\n  text-decoration: none;\n  background-color: #f5f5f5;\n}\na.list-group-item.active,\na.list-group-item.active:hover,\na.list-group-item.active:focus {\n  z-index: 2;\n  color: #fff;\n  background-color: #428bca;\n  border-color: #428bca;\n}\na.list-group-item.active .list-group-item-heading,\na.list-group-item.active:hover .list-group-item-heading,\na.list-group-item.active:focus .list-group-item-heading {\n  color: inherit;\n}\na.list-group-item.active .list-group-item-text,\na.list-group-item.active:hover .list-group-item-text,\na.list-group-item.active:focus .list-group-item-text {\n  color: #e1edf7;\n}\n.list-group-item-success {\n  color: #3c763d;\n  background-color: #dff0d8;\n}\na.list-group-item-success {\n  color: #3c763d;\n}\na.list-group-item-success .list-group-item-heading {\n  color: inherit;\n}\na.list-group-item-success:hover,\na.list-group-item-success:focus {\n  color: #3c763d;\n  background-color: #d0e9c6;\n}\na.list-group-item-success.active,\na.list-group-item-success.active:hover,\na.list-group-item-success.active:focus {\n  color: #fff;\n  background-color: #3c763d;\n  border-color: #3c763d;\n}\n.list-group-item-info {\n  color: #31708f;\n  background-color: #d9edf7;\n}\na.list-group-item-info {\n  color: #31708f;\n}\na.list-group-item-info .list-group-item-heading {\n  color: inherit;\n}\na.list-group-item-info:hover,\na.list-group-item-info:focus {\n  color: #31708f;\n  background-color: #c4e3f3;\n}\na.list-group-item-info.active,\na.list-group-item-info.active:hover,\na.list-group-item-info.active:focus {\n  color: #fff;\n  background-color: #31708f;\n  border-color: #31708f;\n}\n.list-group-item-warning {\n  color: #8a6d3b;\n  background-color: #fcf8e3;\n}\na.list-group-item-warning {\n  color: #8a6d3b;\n}\na.list-group-item-warning .list-group-item-heading {\n  color: inherit;\n}\na.list-group-item-warning:hover,\na.list-group-item-warning:focus {\n  color: #8a6d3b;\n  background-color: #faf2cc;\n}\na.list-group-item-warning.active,\na.list-group-item-warning.active:hover,\na.list-group-item-warning.active:focus {\n  color: #fff;\n  background-color: #8a6d3b;\n  border-color: #8a6d3b;\n}\n.list-group-item-danger {\n  color: #a94442;\n  background-color: #f2dede;\n}\na.list-group-item-danger {\n  color: #a94442;\n}\na.list-group-item-danger .list-group-item-heading {\n  color: inherit;\n}\na.list-group-item-danger:hover,\na.list-group-item-danger:focus {\n  color: #a94442;\n  background-color: #ebcccc;\n}\na.list-group-item-danger.active,\na.list-group-item-danger.active:hover,\na.list-group-item-danger.active:focus {\n  color: #fff;\n  background-color: #a94442;\n  border-color: #a94442;\n}\n.list-group-item-heading {\n  margin-top: 0;\n  margin-bottom: 5px;\n}\n.list-group-item-text {\n  margin-bottom: 0;\n  line-height: 1.3;\n}\n.panel {\n  margin-bottom: 20px;\n  background-color: #fff;\n  border: 1px solid transparent;\n  border-radius: 4px;\n  -webkit-box-shadow: 0 1px 1px rgba(0, 0, 0, .05);\n          box-shadow: 0 1px 1px rgba(0, 0, 0, .05);\n}\n.panel-body {\n  padding: 15px;\n}\n.panel-heading {\n  padding: 10px 15px;\n  border-bottom: 1px solid transparent;\n  border-top-left-radius: 3px;\n  border-top-right-radius: 3px;\n}\n.panel-heading > .dropdown .dropdown-toggle {\n  color: inherit;\n}\n.panel-title {\n  margin-top: 0;\n  margin-bottom: 0;\n  font-size: 16px;\n  color: inherit;\n}\n.panel-title > a {\n  color: inherit;\n}\n.panel-footer {\n  padding: 10px 15px;\n  background-color: #f5f5f5;\n  border-top: 1px solid #ddd;\n  border-bottom-right-radius: 3px;\n  border-bottom-left-radius: 3px;\n}\n.panel > .list-group {\n  margin-bottom: 0;\n}\n.panel > .list-group .list-group-item {\n  border-width: 1px 0;\n  border-radius: 0;\n}\n.panel > .list-group:first-child .list-group-item:first-child {\n  border-top: 0;\n  border-top-left-radius: 3px;\n  border-top-right-radius: 3px;\n}\n.panel > .list-group:last-child .list-group-item:last-child {\n  border-bottom: 0;\n  border-bottom-right-radius: 3px;\n  border-bottom-left-radius: 3px;\n}\n.panel-heading + .list-group .list-group-item:first-child {\n  border-top-width: 0;\n}\n.panel > .table,\n.panel > .table-responsive > .table {\n  margin-bottom: 0;\n}\n.panel > .table:first-child,\n.panel > .table-responsive:first-child > .table:first-child {\n  border-top-left-radius: 3px;\n  border-top-right-radius: 3px;\n}\n.panel > .table:first-child > thead:first-child > tr:first-child td:first-child,\n.panel > .table-responsive:first-child > .table:first-child > thead:first-child > tr:first-child td:first-child,\n.panel > .table:first-child > tbody:first-child > tr:first-child td:first-child,\n.panel > .table-responsive:first-child > .table:first-child > tbody:first-child > tr:first-child td:first-child,\n.panel > .table:first-child > thead:first-child > tr:first-child th:first-child,\n.panel > .table-responsive:first-child > .table:first-child > thead:first-child > tr:first-child th:first-child,\n.panel > .table:first-child > tbody:first-child > tr:first-child th:first-child,\n.panel > .table-responsive:first-child > .table:first-child > tbody:first-child > tr:first-child th:first-child {\n  border-top-left-radius: 3px;\n}\n.panel > .table:first-child > thead:first-child > tr:first-child td:last-child,\n.panel > .table-responsive:first-child > .table:first-child > thead:first-child > tr:first-child td:last-child,\n.panel > .table:first-child > tbody:first-child > tr:first-child td:last-child,\n.panel > .table-responsive:first-child > .table:first-child > tbody:first-child > tr:first-child td:last-child,\n.panel > .table:first-child > thead:first-child > tr:first-child th:last-child,\n.panel > .table-responsive:first-child > .table:first-child > thead:first-child > tr:first-child th:last-child,\n.panel > .table:first-child > tbody:first-child > tr:first-child th:last-child,\n.panel > .table-responsive:first-child > .table:first-child > tbody:first-child > tr:first-child th:last-child {\n  border-top-right-radius: 3px;\n}\n.panel > .table:last-child,\n.panel > .table-responsive:last-child > .table:last-child {\n  border-bottom-right-radius: 3px;\n  border-bottom-left-radius: 3px;\n}\n.panel > .table:last-child > tbody:last-child > tr:last-child td:first-child,\n.panel > .table-responsive:last-child > .table:last-child > tbody:last-child > tr:last-child td:first-child,\n.panel > .table:last-child > tfoot:last-child > tr:last-child td:first-child,\n.panel > .table-responsive:last-child > .table:last-child > tfoot:last-child > tr:last-child td:first-child,\n.panel > .table:last-child > tbody:last-child > tr:last-child th:first-child,\n.panel > .table-responsive:last-child > .table:last-child > tbody:last-child > tr:last-child th:first-child,\n.panel > .table:last-child > tfoot:last-child > tr:last-child th:first-child,\n.panel > .table-responsive:last-child > .table:last-child > tfoot:last-child > tr:last-child th:first-child {\n  border-bottom-left-radius: 3px;\n}\n.panel > .table:last-child > tbody:last-child > tr:last-child td:last-child,\n.panel > .table-responsive:last-child > .table:last-child > tbody:last-child > tr:last-child td:last-child,\n.panel > .table:last-child > tfoot:last-child > tr:last-child td:last-child,\n.panel > .table-responsive:last-child > .table:last-child > tfoot:last-child > tr:last-child td:last-child,\n.panel > .table:last-child > tbody:last-child > tr:last-child th:last-child,\n.panel > .table-responsive:last-child > .table:last-child > tbody:last-child > tr:last-child th:last-child,\n.panel > .table:last-child > tfoot:last-child > tr:last-child th:last-child,\n.panel > .table-responsive:last-child > .table:last-child > tfoot:last-child > tr:last-child th:last-child {\n  border-bottom-right-radius: 3px;\n}\n.panel > .panel-body + .table,\n.panel > .panel-body + .table-responsive {\n  border-top: 1px solid #ddd;\n}\n.panel > .table > tbody:first-child > tr:first-child th,\n.panel > .table > tbody:first-child > tr:first-child td {\n  border-top: 0;\n}\n.panel > .table-bordered,\n.panel > .table-responsive > .table-bordered {\n  border: 0;\n}\n.panel > .table-bordered > thead > tr > th:first-child,\n.panel > .table-responsive > .table-bordered > thead > tr > th:first-child,\n.panel > .table-bordered > tbody > tr > th:first-child,\n.panel > .table-responsive > .table-bordered > tbody > tr > th:first-child,\n.panel > .table-bordered > tfoot > tr > th:first-child,\n.panel > .table-responsive > .table-bordered > tfoot > tr > th:first-child,\n.panel > .table-bordered > thead > tr > td:first-child,\n.panel > .table-responsive > .table-bordered > thead > tr > td:first-child,\n.panel > .table-bordered > tbody > tr > td:first-child,\n.panel > .table-responsive > .table-bordered > tbody > tr > td:first-child,\n.panel > .table-bordered > tfoot > tr > td:first-child,\n.panel > .table-responsive > .table-bordered > tfoot > tr > td:first-child {\n  border-left: 0;\n}\n.panel > .table-bordered > thead > tr > th:last-child,\n.panel > .table-responsive > .table-bordered > thead > tr > th:last-child,\n.panel > .table-bordered > tbody > tr > th:last-child,\n.panel > .table-responsive > .table-bordered > tbody > tr > th:last-child,\n.panel > .table-bordered > tfoot > tr > th:last-child,\n.panel > .table-responsive > .table-bordered > tfoot > tr > th:last-child,\n.panel > .table-bordered > thead > tr > td:last-child,\n.panel > .table-responsive > .table-bordered > thead > tr > td:last-child,\n.panel > .table-bordered > tbody > tr > td:last-child,\n.panel > .table-responsive > .table-bordered > tbody > tr > td:last-child,\n.panel > .table-bordered > tfoot > tr > td:last-child,\n.panel > .table-responsive > .table-bordered > tfoot > tr > td:last-child {\n  border-right: 0;\n}\n.panel > .table-bordered > thead > tr:first-child > td,\n.panel > .table-responsive > .table-bordered > thead > tr:first-child > td,\n.panel > .table-bordered > tbody > tr:first-child > td,\n.panel > .table-responsive > .table-bordered > tbody > tr:first-child > td,\n.panel > .table-bordered > thead > tr:first-child > th,\n.panel > .table-responsive > .table-bordered > thead > tr:first-child > th,\n.panel > .table-bordered > tbody > tr:first-child > th,\n.panel > .table-responsive > .table-bordered > tbody > tr:first-child > th {\n  border-bottom: 0;\n}\n.panel > .table-bordered > tbody > tr:last-child > td,\n.panel > .table-responsive > .table-bordered > tbody > tr:last-child > td,\n.panel > .table-bordered > tfoot > tr:last-child > td,\n.panel > .table-responsive > .table-bordered > tfoot > tr:last-child > td,\n.panel > .table-bordered > tbody > tr:last-child > th,\n.panel > .table-responsive > .table-bordered > tbody > tr:last-child > th,\n.panel > .table-bordered > tfoot > tr:last-child > th,\n.panel > .table-responsive > .table-bordered > tfoot > tr:last-child > th {\n  border-bottom: 0;\n}\n.panel > .table-responsive {\n  margin-bottom: 0;\n  border: 0;\n}\n.panel-group {\n  margin-bottom: 20px;\n}\n.panel-group .panel {\n  margin-bottom: 0;\n  overflow: hidden;\n  border-radius: 4px;\n}\n.panel-group .panel + .panel {\n  margin-top: 5px;\n}\n.panel-group .panel-heading {\n  border-bottom: 0;\n}\n.panel-group .panel-heading + .panel-collapse .panel-body {\n  border-top: 1px solid #ddd;\n}\n.panel-group .panel-footer {\n  border-top: 0;\n}\n.panel-group .panel-footer + .panel-collapse .panel-body {\n  border-bottom: 1px solid #ddd;\n}\n.panel-default {\n  border-color: #ddd;\n}\n.panel-default > .panel-heading {\n  color: #333;\n  background-color: #f5f5f5;\n  border-color: #ddd;\n}\n.panel-default > .panel-heading + .panel-collapse .panel-body {\n  border-top-color: #ddd;\n}\n.panel-default > .panel-footer + .panel-collapse .panel-body {\n  border-bottom-color: #ddd;\n}\n.panel-primary {\n  border-color: #428bca;\n}\n.panel-primary > .panel-heading {\n  color: #fff;\n  background-color: #428bca;\n  border-color: #428bca;\n}\n.panel-primary > .panel-heading + .panel-collapse .panel-body {\n  border-top-color: #428bca;\n}\n.panel-primary > .panel-footer + .panel-collapse .panel-body {\n  border-bottom-color: #428bca;\n}\n.panel-success {\n  border-color: #d6e9c6;\n}\n.panel-success > .panel-heading {\n  color: #3c763d;\n  background-color: #dff0d8;\n  border-color: #d6e9c6;\n}\n.panel-success > .panel-heading + .panel-collapse .panel-body {\n  border-top-color: #d6e9c6;\n}\n.panel-success > .panel-footer + .panel-collapse .panel-body {\n  border-bottom-color: #d6e9c6;\n}\n.panel-info {\n  border-color: #bce8f1;\n}\n.panel-info > .panel-heading {\n  color: #31708f;\n  background-color: #d9edf7;\n  border-color: #bce8f1;\n}\n.panel-info > .panel-heading + .panel-collapse .panel-body {\n  border-top-color: #bce8f1;\n}\n.panel-info > .panel-footer + .panel-collapse .panel-body {\n  border-bottom-color: #bce8f1;\n}\n.panel-warning {\n  border-color: #faebcc;\n}\n.panel-warning > .panel-heading {\n  color: #8a6d3b;\n  background-color: #fcf8e3;\n  border-color: #faebcc;\n}\n.panel-warning > .panel-heading + .panel-collapse .panel-body {\n  border-top-color: #faebcc;\n}\n.panel-warning > .panel-footer + .panel-collapse .panel-body {\n  border-bottom-color: #faebcc;\n}\n.panel-danger {\n  border-color: #ebccd1;\n}\n.panel-danger > .panel-heading {\n  color: #a94442;\n  background-color: #f2dede;\n  border-color: #ebccd1;\n}\n.panel-danger > .panel-heading + .panel-collapse .panel-body {\n  border-top-color: #ebccd1;\n}\n.panel-danger > .panel-footer + .panel-collapse .panel-body {\n  border-bottom-color: #ebccd1;\n}\n.well {\n  min-height: 20px;\n  padding: 19px;\n  margin-bottom: 20px;\n  background-color: #f5f5f5;\n  border: 1px solid #e3e3e3;\n  border-radius: 4px;\n  -webkit-box-shadow: inset 0 1px 1px rgba(0, 0, 0, .05);\n          box-shadow: inset 0 1px 1px rgba(0, 0, 0, .05);\n}\n.well blockquote {\n  border-color: #ddd;\n  border-color: rgba(0, 0, 0, .15);\n}\n.well-lg {\n  padding: 24px;\n  border-radius: 6px;\n}\n.well-sm {\n  padding: 9px;\n  border-radius: 3px;\n}\n.close {\n  float: right;\n  font-size: 21px;\n  font-weight: bold;\n  line-height: 1;\n  color: #000;\n  text-shadow: 0 1px 0 #fff;\n  filter: alpha(opacity=20);\n  opacity: .2;\n}\n.close:hover,\n.close:focus {\n  color: #000;\n  text-decoration: none;\n  cursor: pointer;\n  filter: alpha(opacity=50);\n  opacity: .5;\n}\nbutton.close {\n  -webkit-appearance: none;\n  padding: 0;\n  cursor: pointer;\n  background: transparent;\n  border: 0;\n}\n.modal-open {\n  overflow: hidden;\n}\n.modal {\n  position: fixed;\n  top: 0;\n  right: 0;\n  bottom: 0;\n  left: 0;\n  z-index: 1050;\n  display: none;\n  overflow: auto;\n  overflow-y: scroll;\n  -webkit-overflow-scrolling: touch;\n  outline: 0;\n}\n.modal.fade .modal-dialog {\n  -webkit-transition: -webkit-transform .3s ease-out;\n     -moz-transition:    -moz-transform .3s ease-out;\n       -o-transition:      -o-transform .3s ease-out;\n          transition:         transform .3s ease-out;\n  -webkit-transform: translate(0, -25%);\n      -ms-transform: translate(0, -25%);\n          transform: translate(0, -25%);\n}\n.modal.in .modal-dialog {\n  -webkit-transform: translate(0, 0);\n      -ms-transform: translate(0, 0);\n          transform: translate(0, 0);\n}\n.modal-dialog {\n  position: relative;\n  width: auto;\n  margin: 10px;\n}\n.modal-content {\n  position: relative;\n  background-color: #fff;\n  background-clip: padding-box;\n  border: 1px solid #999;\n  border: 1px solid rgba(0, 0, 0, .2);\n  border-radius: 6px;\n  outline: none;\n  -webkit-box-shadow: 0 3px 9px rgba(0, 0, 0, .5);\n          box-shadow: 0 3px 9px rgba(0, 0, 0, .5);\n}\n.modal-backdrop {\n  position: fixed;\n  top: 0;\n  right: 0;\n  bottom: 0;\n  left: 0;\n  z-index: 1040;\n  background-color: #000;\n}\n.modal-backdrop.fade {\n  filter: alpha(opacity=0);\n  opacity: 0;\n}\n.modal-backdrop.in {\n  filter: alpha(opacity=50);\n  opacity: .5;\n}\n.modal-header {\n  min-height: 16.42857143px;\n  padding: 15px;\n  border-bottom: 1px solid #e5e5e5;\n}\n.modal-header .close {\n  margin-top: -2px;\n}\n.modal-title {\n  margin: 0;\n  line-height: 1.42857143;\n}\n.modal-body {\n  position: relative;\n  padding: 20px;\n}\n.modal-footer {\n  padding: 19px 20px 20px;\n  margin-top: 15px;\n  text-align: right;\n  border-top: 1px solid #e5e5e5;\n}\n.modal-footer .btn + .btn {\n  margin-bottom: 0;\n  margin-left: 5px;\n}\n.modal-footer .btn-group .btn + .btn {\n  margin-left: -1px;\n}\n.modal-footer .btn-block + .btn-block {\n  margin-left: 0;\n}\n@media (min-width: 768px) {\n  .modal-dialog {\n    width: 600px;\n    margin: 30px auto;\n  }\n  .modal-content {\n    -webkit-box-shadow: 0 5px 15px rgba(0, 0, 0, .5);\n            box-shadow: 0 5px 15px rgba(0, 0, 0, .5);\n  }\n  .modal-sm {\n    width: 300px;\n  }\n}\n@media (min-width: 992px) {\n  .modal-lg {\n    width: 900px;\n  }\n}\n.tooltip {\n  position: absolute;\n  z-index: 1030;\n  display: block;\n  font-size: 12px;\n  line-height: 1.4;\n  visibility: visible;\n  filter: alpha(opacity=0);\n  opacity: 0;\n}\n.tooltip.in {\n  filter: alpha(opacity=90);\n  opacity: .9;\n}\n.tooltip.top {\n  padding: 5px 0;\n  margin-top: -3px;\n}\n.tooltip.right {\n  padding: 0 5px;\n  margin-left: 3px;\n}\n.tooltip.bottom {\n  padding: 5px 0;\n  margin-top: 3px;\n}\n.tooltip.left {\n  padding: 0 5px;\n  margin-left: -3px;\n}\n.tooltip-inner {\n  max-width: 200px;\n  padding: 3px 8px;\n  color: #fff;\n  text-align: center;\n  text-decoration: none;\n  background-color: #000;\n  border-radius: 4px;\n}\n.tooltip-arrow {\n  position: absolute;\n  width: 0;\n  height: 0;\n  border-color: transparent;\n  border-style: solid;\n}\n.tooltip.top .tooltip-arrow {\n  bottom: 0;\n  left: 50%;\n  margin-left: -5px;\n  border-width: 5px 5px 0;\n  border-top-color: #000;\n}\n.tooltip.top-left .tooltip-arrow {\n  bottom: 0;\n  left: 5px;\n  border-width: 5px 5px 0;\n  border-top-color: #000;\n}\n.tooltip.top-right .tooltip-arrow {\n  right: 5px;\n  bottom: 0;\n  border-width: 5px 5px 0;\n  border-top-color: #000;\n}\n.tooltip.right .tooltip-arrow {\n  top: 50%;\n  left: 0;\n  margin-top: -5px;\n  border-width: 5px 5px 5px 0;\n  border-right-color: #000;\n}\n.tooltip.left .tooltip-arrow {\n  top: 50%;\n  right: 0;\n  margin-top: -5px;\n  border-width: 5px 0 5px 5px;\n  border-left-color: #000;\n}\n.tooltip.bottom .tooltip-arrow {\n  top: 0;\n  left: 50%;\n  margin-left: -5px;\n  border-width: 0 5px 5px;\n  border-bottom-color: #000;\n}\n.tooltip.bottom-left .tooltip-arrow {\n  top: 0;\n  left: 5px;\n  border-width: 0 5px 5px;\n  border-bottom-color: #000;\n}\n.tooltip.bottom-right .tooltip-arrow {\n  top: 0;\n  right: 5px;\n  border-width: 0 5px 5px;\n  border-bottom-color: #000;\n}\n.popover {\n  position: absolute;\n  top: 0;\n  left: 0;\n  z-index: 1010;\n  display: none;\n  max-width: 276px;\n  padding: 1px;\n  text-align: left;\n  white-space: normal;\n  background-color: #fff;\n  background-clip: padding-box;\n  border: 1px solid #ccc;\n  border: 1px solid rgba(0, 0, 0, .2);\n  border-radius: 6px;\n  -webkit-box-shadow: 0 5px 10px rgba(0, 0, 0, .2);\n          box-shadow: 0 5px 10px rgba(0, 0, 0, .2);\n}\n.popover.top {\n  margin-top: -10px;\n}\n.popover.right {\n  margin-left: 10px;\n}\n.popover.bottom {\n  margin-top: 10px;\n}\n.popover.left {\n  margin-left: -10px;\n}\n.popover-title {\n  padding: 8px 14px;\n  margin: 0;\n  font-size: 14px;\n  font-weight: normal;\n  line-height: 18px;\n  background-color: #f7f7f7;\n  border-bottom: 1px solid #ebebeb;\n  border-radius: 5px 5px 0 0;\n}\n.popover-content {\n  padding: 9px 14px;\n}\n.popover > .arrow,\n.popover > .arrow:after {\n  position: absolute;\n  display: block;\n  width: 0;\n  height: 0;\n  border-color: transparent;\n  border-style: solid;\n}\n.popover > .arrow {\n  border-width: 11px;\n}\n.popover > .arrow:after {\n  content: \"\";\n  border-width: 10px;\n}\n.popover.top > .arrow {\n  bottom: -11px;\n  left: 50%;\n  margin-left: -11px;\n  border-top-color: #999;\n  border-top-color: rgba(0, 0, 0, .25);\n  border-bottom-width: 0;\n}\n.popover.top > .arrow:after {\n  bottom: 1px;\n  margin-left: -10px;\n  content: \" \";\n  border-top-color: #fff;\n  border-bottom-width: 0;\n}\n.popover.right > .arrow {\n  top: 50%;\n  left: -11px;\n  margin-top: -11px;\n  border-right-color: #999;\n  border-right-color: rgba(0, 0, 0, .25);\n  border-left-width: 0;\n}\n.popover.right > .arrow:after {\n  bottom: -10px;\n  left: 1px;\n  content: \" \";\n  border-right-color: #fff;\n  border-left-width: 0;\n}\n.popover.bottom > .arrow {\n  top: -11px;\n  left: 50%;\n  margin-left: -11px;\n  border-top-width: 0;\n  border-bottom-color: #999;\n  border-bottom-color: rgba(0, 0, 0, .25);\n}\n.popover.bottom > .arrow:after {\n  top: 1px;\n  margin-left: -10px;\n  content: \" \";\n  border-top-width: 0;\n  border-bottom-color: #fff;\n}\n.popover.left > .arrow {\n  top: 50%;\n  right: -11px;\n  margin-top: -11px;\n  border-right-width: 0;\n  border-left-color: #999;\n  border-left-color: rgba(0, 0, 0, .25);\n}\n.popover.left > .arrow:after {\n  right: 1px;\n  bottom: -10px;\n  content: \" \";\n  border-right-width: 0;\n  border-left-color: #fff;\n}\n.carousel {\n  position: relative;\n}\n.carousel-inner {\n  position: relative;\n  width: 100%;\n  overflow: hidden;\n}\n.carousel-inner > .item {\n  position: relative;\n  display: none;\n  -webkit-transition: .6s ease-in-out left;\n          transition: .6s ease-in-out left;\n}\n.carousel-inner > .item > img,\n.carousel-inner > .item > a > img {\n  line-height: 1;\n}\n.carousel-inner > .active,\n.carousel-inner > .next,\n.carousel-inner > .prev {\n  display: block;\n}\n.carousel-inner > .active {\n  left: 0;\n}\n.carousel-inner > .next,\n.carousel-inner > .prev {\n  position: absolute;\n  top: 0;\n  width: 100%;\n}\n.carousel-inner > .next {\n  left: 100%;\n}\n.carousel-inner > .prev {\n  left: -100%;\n}\n.carousel-inner > .next.left,\n.carousel-inner > .prev.right {\n  left: 0;\n}\n.carousel-inner > .active.left {\n  left: -100%;\n}\n.carousel-inner > .active.right {\n  left: 100%;\n}\n.carousel-control {\n  position: absolute;\n  top: 0;\n  bottom: 0;\n  left: 0;\n  width: 15%;\n  font-size: 20px;\n  color: #fff;\n  text-align: center;\n  text-shadow: 0 1px 2px rgba(0, 0, 0, .6);\n  filter: alpha(opacity=50);\n  opacity: .5;\n}\n.carousel-control.left {\n  background-image: -webkit-linear-gradient(left, color-stop(rgba(0, 0, 0, .5) 0%), color-stop(rgba(0, 0, 0, .0001) 100%));\n  background-image:         linear-gradient(to right, rgba(0, 0, 0, .5) 0%, rgba(0, 0, 0, .0001) 100%);\n  filter: progid:DXImageTransform.Microsoft.gradient(startColorstr='#80000000', endColorstr='#00000000', GradientType=1);\n  background-repeat: repeat-x;\n}\n.carousel-control.right {\n  right: 0;\n  left: auto;\n  background-image: -webkit-linear-gradient(left, color-stop(rgba(0, 0, 0, .0001) 0%), color-stop(rgba(0, 0, 0, .5) 100%));\n  background-image:         linear-gradient(to right, rgba(0, 0, 0, .0001) 0%, rgba(0, 0, 0, .5) 100%);\n  filter: progid:DXImageTransform.Microsoft.gradient(startColorstr='#00000000', endColorstr='#80000000', GradientType=1);\n  background-repeat: repeat-x;\n}\n.carousel-control:hover,\n.carousel-control:focus {\n  color: #fff;\n  text-decoration: none;\n  filter: alpha(opacity=90);\n  outline: none;\n  opacity: .9;\n}\n.carousel-control .icon-prev,\n.carousel-control .icon-next,\n.carousel-control .glyphicon-chevron-left,\n.carousel-control .glyphicon-chevron-right {\n  position: absolute;\n  top: 50%;\n  z-index: 5;\n  display: inline-block;\n}\n.carousel-control .icon-prev,\n.carousel-control .glyphicon-chevron-left {\n  left: 50%;\n}\n.carousel-control .icon-next,\n.carousel-control .glyphicon-chevron-right {\n  right: 50%;\n}\n.carousel-control .icon-prev,\n.carousel-control .icon-next {\n  width: 20px;\n  height: 20px;\n  margin-top: -10px;\n  margin-left: -10px;\n  font-family: serif;\n}\n.carousel-control .icon-prev:before {\n  content: '\\2039';\n}\n.carousel-control .icon-next:before {\n  content: '\\203a';\n}\n.carousel-indicators {\n  position: absolute;\n  bottom: 10px;\n  left: 50%;\n  z-index: 15;\n  width: 60%;\n  padding-left: 0;\n  margin-left: -30%;\n  text-align: center;\n  list-style: none;\n}\n.carousel-indicators li {\n  display: inline-block;\n  width: 10px;\n  height: 10px;\n  margin: 1px;\n  text-indent: -999px;\n  cursor: pointer;\n  background-color: #000 \\9;\n  background-color: rgba(0, 0, 0, 0);\n  border: 1px solid #fff;\n  border-radius: 10px;\n}\n.carousel-indicators .active {\n  width: 12px;\n  height: 12px;\n  margin: 0;\n  background-color: #fff;\n}\n.carousel-caption {\n  position: absolute;\n  right: 15%;\n  bottom: 20px;\n  left: 15%;\n  z-index: 10;\n  padding-top: 20px;\n  padding-bottom: 20px;\n  color: #fff;\n  text-align: center;\n  text-shadow: 0 1px 2px rgba(0, 0, 0, .6);\n}\n.carousel-caption .btn {\n  text-shadow: none;\n}\n@media screen and (min-width: 768px) {\n  .carousel-control .glyphicon-chevron-left,\n  .carousel-control .glyphicon-chevron-right,\n  .carousel-control .icon-prev,\n  .carousel-control .icon-next {\n    width: 30px;\n    height: 30px;\n    margin-top: -15px;\n    margin-left: -15px;\n    font-size: 30px;\n  }\n  .carousel-caption {\n    right: 20%;\n    left: 20%;\n    padding-bottom: 30px;\n  }\n  .carousel-indicators {\n    bottom: 20px;\n  }\n}\n.clearfix:before,\n.clearfix:after,\n.container:before,\n.container:after,\n.container-fluid:before,\n.container-fluid:after,\n.row:before,\n.row:after,\n.form-horizontal .form-group:before,\n.form-horizontal .form-group:after,\n.btn-toolbar:before,\n.btn-toolbar:after,\n.btn-group-vertical > .btn-group:before,\n.btn-group-vertical > .btn-group:after,\n.nav:before,\n.nav:after,\n.navbar:before,\n.navbar:after,\n.navbar-header:before,\n.navbar-header:after,\n.navbar-collapse:before,\n.navbar-collapse:after,\n.pager:before,\n.pager:after,\n.panel-body:before,\n.panel-body:after,\n.modal-footer:before,\n.modal-footer:after {\n  display: table;\n  content: \" \";\n}\n.clearfix:after,\n.container:after,\n.container-fluid:after,\n.row:after,\n.form-horizontal .form-group:after,\n.btn-toolbar:after,\n.btn-group-vertical > .btn-group:after,\n.nav:after,\n.navbar:after,\n.navbar-header:after,\n.navbar-collapse:after,\n.pager:after,\n.panel-body:after,\n.modal-footer:after {\n  clear: both;\n}\n.center-block {\n  display: block;\n  margin-right: auto;\n  margin-left: auto;\n}\n.pull-right {\n  float: right !important;\n}\n.pull-left {\n  float: left !important;\n}\n.hide {\n  display: none !important;\n}\n.show {\n  display: block !important;\n}\n.invisible {\n  visibility: hidden;\n}\n.text-hide {\n  font: 0/0 a;\n  color: transparent;\n  text-shadow: none;\n  background-color: transparent;\n  border: 0;\n}\n.hidden {\n  display: none !important;\n  visibility: hidden !important;\n}\n.affix {\n  position: fixed;\n}\n@-ms-viewport {\n  width: device-width;\n}\n.visible-xs,\n.visible-sm,\n.visible-md,\n.visible-lg {\n  display: none !important;\n}\n@media (max-width: 767px) {\n  .visible-xs {\n    display: block !important;\n  }\n  table.visible-xs {\n    display: table;\n  }\n  tr.visible-xs {\n    display: table-row !important;\n  }\n  th.visible-xs,\n  td.visible-xs {\n    display: table-cell !important;\n  }\n}\n@media (min-width: 768px) and (max-width: 991px) {\n  .visible-sm {\n    display: block !important;\n  }\n  table.visible-sm {\n    display: table;\n  }\n  tr.visible-sm {\n    display: table-row !important;\n  }\n  th.visible-sm,\n  td.visible-sm {\n    display: table-cell !important;\n  }\n}\n@media (min-width: 992px) and (max-width: 1199px) {\n  .visible-md {\n    display: block !important;\n  }\n  table.visible-md {\n    display: table;\n  }\n  tr.visible-md {\n    display: table-row !important;\n  }\n  th.visible-md,\n  td.visible-md {\n    display: table-cell !important;\n  }\n}\n@media (min-width: 1200px) {\n  .visible-lg {\n    display: block !important;\n  }\n  table.visible-lg {\n    display: table;\n  }\n  tr.visible-lg {\n    display: table-row !important;\n  }\n  th.visible-lg,\n  td.visible-lg {\n    display: table-cell !important;\n  }\n}\n@media (max-width: 767px) {\n  .hidden-xs {\n    display: none !important;\n  }\n}\n@media (min-width: 768px) and (max-width: 991px) {\n  .hidden-sm {\n    display: none !important;\n  }\n}\n@media (min-width: 992px) and (max-width: 1199px) {\n  .hidden-md {\n    display: none !important;\n  }\n}\n@media (min-width: 1200px) {\n  .hidden-lg {\n    display: none !important;\n  }\n}\n.visible-print {\n  display: none !important;\n}\n@media print {\n  .visible-print {\n    display: block !important;\n  }\n  table.visible-print {\n    display: table;\n  }\n  tr.visible-print {\n    display: table-row !important;\n  }\n  th.visible-print,\n  td.visible-print {\n    display: table-cell !important;\n  }\n}\n@media print {\n  .hidden-print {\n    display: none !important;\n  }\n}\n/*# sourceMappingURL=bootstrap.css.map */\n", error in=w123) -> (refnum out=w126:refnum<file>, error out=w124:errorcluster)  [unwired: 1 in, 1 out]
          n50 = Close File(refnum=w126, error in=w124) -> (error out=→"error out":errorcluster)  [unwired: 1 out]
        }
      }
    }
  }
